vi "MATSYA GUI.vi"() -> ()   [LabVIEW 2018]
uses:
  <vilib>/picture/3D Picture Control/NI_3D Picture Control.lvlib
  179b0847-8d0b-44e4-b652-b0f693d2dd6b.vi
  a317c550-89e4-45e7-94c4-efb925d81c87.vi
  00af5911-90ac-44b2-9784-eceb848f2253.vi
  66d8c7ed-505b-4229-a511-ec78d290ed99.vi
  Host/Controls/Host Data Cluster.ctl
  Main Engine/Controls/Main Engine CPU Info.ctl
panel:
  out "AI":dbl[](array[numeric]) format="%#.6f"
  out "Data Tx/Rx 2":string
  out "output cluster":T1
  out "error out 3":errorcluster
  out "Power  Status":string
  out "USER STRING":string
  out "length":i32
  out "error in (no error) 2":errorcluster
  out "elements in queue":i32
  out "PDE_P 24 Current (A)":dbl caption="PDE_P Current (A)" format="%_3g"
  out "PDE_P 24 Voltage (V) 2":dbl caption="PDE_P Voltage (V)" format="%.1f"
  out "PDE_P 24 Voltage (V)":dbl caption="PDE_P Voltage (V)" format="%.1f"
  out "Slave":bool
  out "error out 2":errorcluster
  out "String":string
  out "Water Ingress":bool caption="AGS 1"
  out "Comm Status":bool caption="AGS 2"
  out "Temp":dbl caption="Displacement"
  out "Battery SOC":dbl caption="Displacement"
  out "CO2":dbl caption="Displacement"
  out "O2":dbl caption="Displacement"
  in  "Quit":bool caption="Power"
  in  "Mode":bool caption="Reset"
  out "Warnings/Alarms":string
  in  "Thrusters \ninterlock":bool
  out "Present Time":string caption="Present Text"
  out "Mission Start Time":string caption="Start Time Text"
  out "Dive #":dbl format="%#_2g"
  in  "Tab Control":T2(tab)
  out "Altitude":dbl(slide)=1.0 scale=0.0..90.0
  out "Depth":dbl(slide)=1.0
  out "Vertical    Speed":dbl format="%#_4g"
  out "Lateral\nSpeed":dbl format="%#.4g"
  out "Forward\nSpeed":dbl format="%#_4g"
  out "Longitude":dbl format="%#_8g"
  out "Latitude":dbl format="%#_8g"
  out "Ship\n Heading":dbl format="%#.4f"
  out "Heading":sgl
  out "Pitch":sgl
  out "Roll":sgl
  out "3D MATSYA":refnum<vi>(3d-picture)
  out "HSSS_S":T3 caption="HSSS_P" {"Oxygen_S" scale=19.0..25.0; "CO2_s" scale=0.0..5000.0; "Temp in Deg C_S" scale=0.0..100.0; "Humidity_S in %" scale=0.0..100.0; "Presssure in mbar_S" scale=800.0..1200.0}
  out "HSSS_P":T4 {"Oxygen_P" scale=19.0..25.0; "CO2_P" scale=0.0..5000.0; "Temp in Deg C_P" scale=0.0..100.0; "Humidity_P in %" scale=0.0..100.0; "Presssure in mbar_P" scale=800.0..1200.0}
  in  "HSSS_P Power":bool
  in  "Dehumidifier_S":bool
  in  "HSSS_S Power":bool
  in  "Co2 Scrubber_P":bool
  in  "Co2 Scrubber_S":bool
  in  "Dehumidifier_P":bool
  out "MBS Air Pressure 2":dbl(slide)=1.0 caption="MBS Air Pressure 1" scale=0.3..300.0
  out "Motor Water Entry":dbl
  out "HP AIR pressure 2":dbl
  out "HP AIR pressure 1":dbl
  out "HPU temp":dbl
  out "HPU Pressure":dbl
  out "MBS JB Water Entry":dbl
  in  "MBS_manual":bool
  in  "VBS SET":dbl
  in  "Trim motor enable":bool
  out "Motor temp":dbl
  out "SUB Pitch":dbl
  out "MBS Air Pressure 1":dbl(slide)=1.0 scale=0.3..300.0
  in  "VBS_Water out":bool
  in  "VBS Water In":bool
  in  "Auto Tim Enable":bool
  out "VBS Tank":dbl(slide)=1.0 scale=0.0..300.0
  in  "VBS_HPU_Enable":bool
  in  "MBS Freeboard":bool
  in  "MBS Desent":bool
  in  "Thrusters_T3":bool
  in  "T3-Signal":bool
  out "T8":T5 {"T8 Temp" format="%#.1f"; "T8 Current" format="%#_2g"; "T8 Voltage" format="%#_3g"; "T8 Speed" scale=0.0..1600.0}
  in  "T8 ctrl":dbl min=-10.0 max=10.0
  out "T6":T6 {"T6 Temp" format="%#.1f"; "T6 Current" format="%#_2g"; "T6 Voltage" format="%#_3g"; "T6 Speed" scale=0.0..1600.0}
  in  "T6 ctrl":dbl min=-10.0 max=10.0
  out "T4":T7 {"T4 Temp" format="%#.1f"; "T4 Current" format="%#_2g"; "T4 Voltage" format="%#_3g"; "T4 Speed" scale=0.0..1600.0}
  in  "T4 ctrl":dbl min=-10.0 max=10.0
  out "T2":T8 {"T2 Temp" format="%#.1f"; "T2 Current" format="%#_2g"; "T2 Voltage" format="%#_3g"; "T2 Speed" scale=0.0..1600.0}
  in  "T2 ctrl":dbl min=-10.0 max=10.0
  in  "T7 ctrl":dbl min=-10.0 max=10.0
  in  "T5 ctrl":dbl min=-10.0 max=10.0
  out "T7":T9 {"T7 Temp" format="%#.1f"; "T7 Current" format="%#_2g"; "T7 Voltage" format="%#_3g"; "T7 Speed" scale=0.0..1600.0}
  out "T5":T10 {"T5 Temp" format="%#.1f"; "T5 Current" format="%#_2g"; "T5 Voltage" format="%#_3g"; "T5 Speed" scale=0.0..1600.0}
  out "T1":T11 {"T1 Temp" format="%#.1f"; "T1 Current" format="%#_2g"; "T1 Voltage" format="%#_3g"; "T1 Speed" scale=0.0..1600.0}
  in  "T3 ctrl":dbl min=-10.0 max=10.0
  in  "T1 ctrl":dbl min=-10.0 max=10.0
  out "T3":T12 {"T3  Temp" format="%#.1f"; "T3 Current" format="%#_2g"; "T3 Voltage" format="%#_3g"; "T3 Speed" scale=0.0..1600.0}
  in  "T2Power":bool
  in  "T4Power":bool
  in  "T6Power":bool
  in  "T8Power":bool
  in  "T3Power":bool
  in  "T5Power":bool
  in  "T7Power":bool
  in  "T1Power":bool
  in  "Thrusters_T1":bool
  in  "T1-Signal":bool
  in  "Thrusters _T5":bool
  in  "T5-Signal":bool
  in  "Thrusters _T7":bool
  in  "T7-Signal":bool
  in  "Thrusters _T2":bool
  in  "T2-Signal":bool
  in  "Thrusters _T4":bool
  in  "T4-Signal":bool
  in  "Thrusters _T6":bool
  in  "T6-Signal":bool
  in  "Thrusters _T8":bool
  in  "T8-Signal":bool
  out "MB_S":T13 {"MB_S Temp (deg C)" format="%_3g"; "MB_S Power (W)" format="%_3f"; "MB_S Current (A)" format="%_3g"; "MB_S Volt (V)" scale=0.0..160.0; "MB_S SOC (%)" format="%_3g"}
  out "MB_P":T14 {"MB_P Temp (deg C)" format="%_3g"; "MB_P Power (W)" format="%_3f"; "MB_P Current (A)" format="%_3g"; "MB_P Volt (V)" scale=100.0..160.0; "MB_P SOC (%)" format="%_3g"}
  out "AUX_S":T15 {"AUX_S Temp (deg C)" format="%_3g"; "AUX_S Power (W)" format="%_3g"; "AUX_S Current (A)" format="%_3g"; "AUX_S Volt (V)" scale=0.0..60.0; "AUX_S SOC (%)" format="%_3g"}
  out "IDE_S":T16 {"IDE_S Temp (degC)" format="%_3g"; "IDE_S Current (A)" format="%_3g"; "IDE_S Voltage (V)" format="%_3g"; "IDE_S IR  (Kohm)" format="%_3f"}
  out "IDE_P":T17 {"IDE_P Temp (degC)" format="%_3g"; "IDE_P Current (A)" format="%_3g"; "IDE_P Voltage (V)" format="%_3g"; "IDE_P IR (kohm)" format="%_3f"}
  out "PDE_S":T18 {"PDE_S Current (A)" format="%_3g"; "PDE_S Temp (degC)" format="%_3g"; "PDE_S Voltage (V)" format="%.1f"; "PDE_S IR (Kohm)" format="%_3f"}
  out "PDE_P":T19 {"PDE_P Temp (degC)" format="%_3g"; "PDE_P Current (A)" format="%_3g"; "PDE_P Voltage (V)" format="%.1f"; "PDE_P IR (Kohm)" format="%_3f"}
  out "AUX_P":T20 {"AUX_P Temp (deg C)" format="%_3g"; "AUX_P Power (W)" format="%_3g"; "AUX_P Current (A)" format="%_3g"; "AUX_P Volt (V)" scale=0.0..40.0; "AUX_P SOC (%)" format="%_3g"}
  in  "HYD_OIL":bool
  in  "ALTITUDE":bool
  in  "DEPTH":bool
  in  "AB_P":bool
  in  "AB_S":bool
  in  "BATS_S":bool
  in  "TJB_S":bool
  in  "PJB_S":bool
  in  "PDE_S":bool
  in  "IDE_S":bool
  in  "PS_S":bool
  in  "MB_S":bool
  in  "PDE_148_S":bool
  in  "PDE_S":bool
  in  "IDE_S":bool
  in  "EB_S":bool
  in  "UB_S":bool
  in  "MB_P":bool
  in  "PDE_148_P":bool
  in  "PDE_P":bool
  in  "IDE_P":bool
  in  "EB_P":bool
  in  "UB_P":bool
  in  "BATS_P":bool
  in  "TJB_P":bool
  in  "PJB_P":bool
  in  "PDE_P":bool
  in  "IDE_P":bool
  in  "PS_P":bool
  out "Hyd oil":bool
  out "Depth":bool
  out "Altitude":bool
  out "PDE 148_S":bool
  out "PDE_S":bool
  out "IDE_S":bool
  out "EB_S":bool
  out "UB_S":bool
  out "AB_S":bool
  out "MB_S":bool
  out "PDE 148_P":bool
  out "PDE_P":bool
  out "IDE_P":bool
  out "EB_P":bool
  out "UB_P":bool
  out "AB_P":bool
  out "MB_P":bool
  out "TJB_S":bool
  out "PJB_S":bool
  out "PDE_S 3":bool
  out "IDE_S 3":bool
  out "PS_S":bool
  out "TJB_P":bool
  out "PJB_P":bool
  out "PDE_P 3":bool
  out "IDE_P 3":bool
  out "PS_P":bool
  out "BATS_S":bool
  out "BATS_P":bool
  in  "Dissolved O2":bool caption="LED Light S4"
  in  "Camera Controls":T21
  in  "Pan and Tilt P2":bool
  in  "148 V LED S3":bool
  in  "148 V LED S4":bool
  in  "148 V LED S1":bool
  in  "148 V LED S2":bool
  in  "LED Light S3":bool
  in  "LED Light S4":bool
  in  "HD Camera S3":bool
  in  "LED Light S2":bool
  in  "SD Camera S4":bool
  in  "HD Camera S1":bool
  in  "HD Camera S2":bool
  in  "4K camera S":bool
  in  "LED Light P3":bool
  in  "LED Light P4":bool
  in  "HD Camera P3":bool
  in  "LED Light P2":bool
  in  "SD_Camera_P4":bool
  in  "HD Camera P1":bool
  in  "HD Camera P2":bool
  in  "4K camera P":bool
  out "ROV PnT Indication":T22 {"TILT" max=120 step=2 scale=-110.0..110.0; "PAN" scale=-150.0..150.0}
  in  "PnT CTRL":T23
  in  "148 V LED P2":bool
  in  "148 V LED P1":bool
  in  "148 V LED P3":bool
  in  "148 V LED P4":bool
  in  "Pan and Tilt S":bool
  in  "Pan and Tilt P1":bool
  in  "Tab Control 2":enum32{"LED 1", "LED 2"}(tab)
  in  "led 1 Dim% (10x)":dbl(slide) caption="Dim% (10x)" min=0.0 max=5.0 step=1.0 scale=0.0..5.0
  in  "led 2 Dim% (10x)":dbl(slide) caption="Dim% (10x)" min=0.0 max=5.0 step=1.0 scale=0.0..5.0
  out "S_Depth":dbl
  out "S_Longitude":dbl
  out "S_Latitude":dbl
  out "S_Heading":dbl
  out "S_Pitch":dbl
  out "S_Roll":dbl
  in  "Dissolved Oxygen":bool
  in  "Trim System":bool
  in  "Plume Detector":bool
  out "Altitude 2":dbl format="%#_4g"
  out "Depth Sensor Sec 2":dbl format="%#_4g"
  out "Depth Sensor Pri 2":dbl format="%#_4g"
  in  "Laser Light 4":bool
  in  "Laser Light 3":bool
  in  "Laser Light 2":bool
  in  "Laser Light 1":bool
  in  "Magnetometer":bool
  in  "Heat Probe Sensor":bool
  in  "CO2 Sensor":bool
  in  "Subbottom Profiler":bool
  in  "Imaging Sonar":bool
  in  "SVP, Turbidity, pH":bool
  in  "Multibeam Sonar":bool
  out "pH":dbl format="%#_4g"
  out "Methane con":dbl format="%#_4g"
  out "Carbon Dioxide":dbl format="%#_4g"
  out "Disolved Oxygen":dbl format="%#_4g"
  in  "Altimeter":bool
  in  "Conduct & Temp":bool
  out "Turbidity":dbl format="%#_4g"
  out "Subea Temp_2":dbl format="%#_4g"
  out "Water Density":dbl format="%#_4g"
  out "Salanity":dbl format="%#_4g"
  in  "INS-DVL":bool
  in  "Depth Sensor Pri":bool
  out "Sound Velocity":dbl format="%#_4g"
  out "Conductivity":dbl format="%#_4g"
  in  "Methane_Sensor":bool
  in  "VBS":bool
  in  "MBS":bool
  out "Error Logging":string[][](table)
  in  "Data log":bool
  in  "Data Logging":dbl(slide) scale=0.0..60.0
  out "Event Logging":string[][](table)
  in  "Channel 2":u16(ring) caption="Ring"
  out "Graph 2":dbl[](graph) caption="Displacement"
  out "Graph 1":dbl[](graph) caption="Displacement"
  in  "Channel":u16(ring) caption="Ring"
  out "BAT VOL 2":dbl(slide)=1.0 scale=100.0..170.0
  out "BAT TEMP 2":dbl(slide)=1.0 scale=0.0..50.0
  out "BAT SOC 2":dbl(slide)=1.0 scale=0.0..200.0
  out "BAT CUR 2":dbl(slide)=1.0 scale=0.0..100.0
  out "BAT VOL":dbl(slide)=1.0 scale=100.0..170.0
  out "BAT TEMP":dbl(slide)=1.0 scale=0.0..50.0
  out "BAT SOC":dbl(slide)=1.0 scale=0.0..200.0
  out "BAT CUR":dbl(slide)=1.0 scale=0.0..100.0
  out "portside 50 Kwh":T24
  out "50 kwh star board":T25
  in  "read/write":bool
  in  "Enum - Menu":enum16{"Low", "Medium", "High", "Very High"}(ring)
  out "Ship Time":sgl caption="Longitude"
  out "Ship Heading":sgl caption="Longitude" format="%#_8g"
  out "Ship Latitude":sgl caption="Latitude" format="%#_9g"
  out "Ship Longitude":sgl caption="Longitude" format="%#_8g"
  in  "Read/ Write":bool
  in  "Data Sending Mode":bool
  out "Modem Ready Status":bool
  out "Data Out":string
  in  "Data Tx/Rx":string
  in  "Byte Count":u32=20
  in  "Crew Status PILOT":bool caption="PILOT"
  in  "Crew StatusCO-PILOT":bool caption="CO-PILOT"
  in  "Crew Status OBSERVER":bool caption="OBSERVER"
  out "Radio Buttons 2":enum32{"Item 0", "Item 1", "Item 2", "Item 3"}(radio)
  in  "Crew Status OBSERVER 2":bool caption="Power"
  in  "Joystick":bool
  in  "Access":bool=TRUE
  out "Quit?":bool
  out "PS_P_Comm_status":bool
  out "PS_S_Comm_Status":bool
  out "PDE_P_Comm_Status":bool
  out "PDE_S_Comm_Status":bool
  out "IDE_P_Comm_Status":bool
  out "IDE_S_Comm_Status":bool
  out "Serial":string[][](array[string])
  out "System Down?":bool
  in  "OIM RESET_S2":bool
  in  "OIM RESET _S1":bool
  in  "BATS_S":bool
  in  "OIM RESET_P2":bool
  in  "OIM RESET _P1":bool
  in  "MBS_P":bool
  in  "LED Light S1":bool
  in  "LED Light P1":bool
  out "TCP - Serial":string[][](array[string])
  in  "error In":errorcluster
  out "PS_P 2":T26
  out "IDE_P 2":T26
  out "PS_S 2":T26
  out "PDE_S 2":T26
  out "PDE_P 2":T26
  out "IDE_S 2":T26
  out "Completed Time":string caption="Elapsed Time Text"
  # "NATIONAL INSTITUTE OF OCEAN TECHNOLOGY\nManned Submersible - MATSYA 6000"
  # "Battery5\n81 Power\n82Current\n83 Pack Voltage\n84ID cell max\n85Max temperature\n86 ID Cell min\n87 Min temperature\n88 Temperature\n89 SOC\n90 SOH\n91 State Bat\n92Flags Bat\n93Fault Code\n94 Level Faults\n95Warnings"
  # "Global Data\n01 Battery Current\n02 Battery Voltage\n03 SOC\n04 SOH\n05 Mean Temperature\n06 Status Faults\n07 Status Warning\n08 Status battery\n\nSummary 10 kW modules\n09 Battery ID\n10 Max temperature\n11 Pack Max voltage\n12 battrey ID Voltgae\n13 Battery ID Min Voltage\n14 Pack Min Voltage\n15 Battery ID min\n16 ID cell Min\n17 Min Cell Voltage\n18 Battery ID Max\n19 ID cell Max\n20 Max cell voltage\n\nEach 10 kW Batteries                                                        \nBattery1\n21 Power\n22 Current\n23 Pack Voltage\n24 ID cell max\n25 Max temperature\n26 ID Cell min\n27 Min temperature\n28 Temperature\n29 SOC\n30 SOH\n31 State Bat\n32 Flags Bat\n33 Fault Code\n34 Level Faults\n35 Warnings\n\nBattery2\n36 Power\n37 Current\n38 Pack Voltage\n39 ID cell max\n40 Max temperature\n41 ID Cell min\n42 Min temperature\n43 Temperature\n44 SOC\n45 SOH\n46 State Bat\n47 Flags Bat\n48 Fault Code\n49 Level Faults\n50 Warnings\n\n\n\nBattery3\n51 Power\n52Current\n53 Pack Voltage\n54 ID cell max\n55Max temperature\n56 ID Cell min\n57 Min temperature\n58 Temperature\n59 SOC\n60 SOH\n61 State Bat\n62 Flags Bat\n63 Fault Code\n64 Level Faults\n65Warnings"
  # "Battery4\n66 Power\n67Current\n68 Pack Voltage\n69ID cell max\n70Max temperature\n71 ID Cell min\n72 Min temperature\n73 Temperature\n74 SOC\n75 SOH\n76 State Bat\n77Flags Bat\n78 Fault Code\n79 Level Faults\n80Warnings"
  # "Comm Status"
  # "N"
  # "deg"
  # "deg"
  # "E"
  # "m/s"
  # "W"
  # "m/s"
  # "m/s"
  # "S"
  # "deg"
  # "m"
  # "m"
  # "deg"
  # "MBS"
  # "VBS"
  # "TRIM"
  # "PDE_P"
  # "T_3"
  # "T_5"
  # "T_7"
  # "T_1"
  # "V"
  # "A"
  # "deg C"
  # "V"
  # "A"
  # "deg C"
  # "V"
  # "A"
  # "deg C"
  # "V"
  # "A"
  # "deg C"
  # "V"
  # "A"
  # "deg C"
  # "V"
  # "A"
  # "deg C"
  # "V"
  # "A"
  # "deg C"
  # "V"
  # "A"
  # "deg C"
  # "IDE_P"
  # "IDE_P"
  # "Insulation_S"
  # "Insulation_P"
  # "Water Ingress_S"
  # "Water Ingress_P"
  # "Underwater Imaging"
  # "deg"
  # "deg"
  # "Deg"
  # "Deg"
  # "Scientific Sensors"
  # "Sec.INS"
  # "Port side"
  # "Starboard"
  # "blow valve 1"
  # "blow valve 2"
  # "Forward"
  # "Reverse"
  # "BATTERY 50 kWh STATUS"
  # "port side"
  # "starboard side"
  # "BAT 1"
  # "BAT 4"
  # "BAT 2"
  # "BAT 3"
  # "BAT 5"
  # "CUR"
  # "VOT"
  # "ID Cell Max"
  # "Max Temp"
  # "ID Cell Min"
  # "Min Temp"
  # "Temp"
  # "SOC"
  # "SOH"
  # "BAT 6"
  # "BAT 7"
  # "BAT 8"
  # "BAT 9"
  # "BAT 10"
  # "CUR"
  # "VOT"
  # "ID Cell Max"
  # "Max Temp"
  # "ID Cell Min"
  # "Min Temp"
  # "Temp"
  # "SOC"
  # "SOH"
  # "Power Status"
  # "Crew Status"
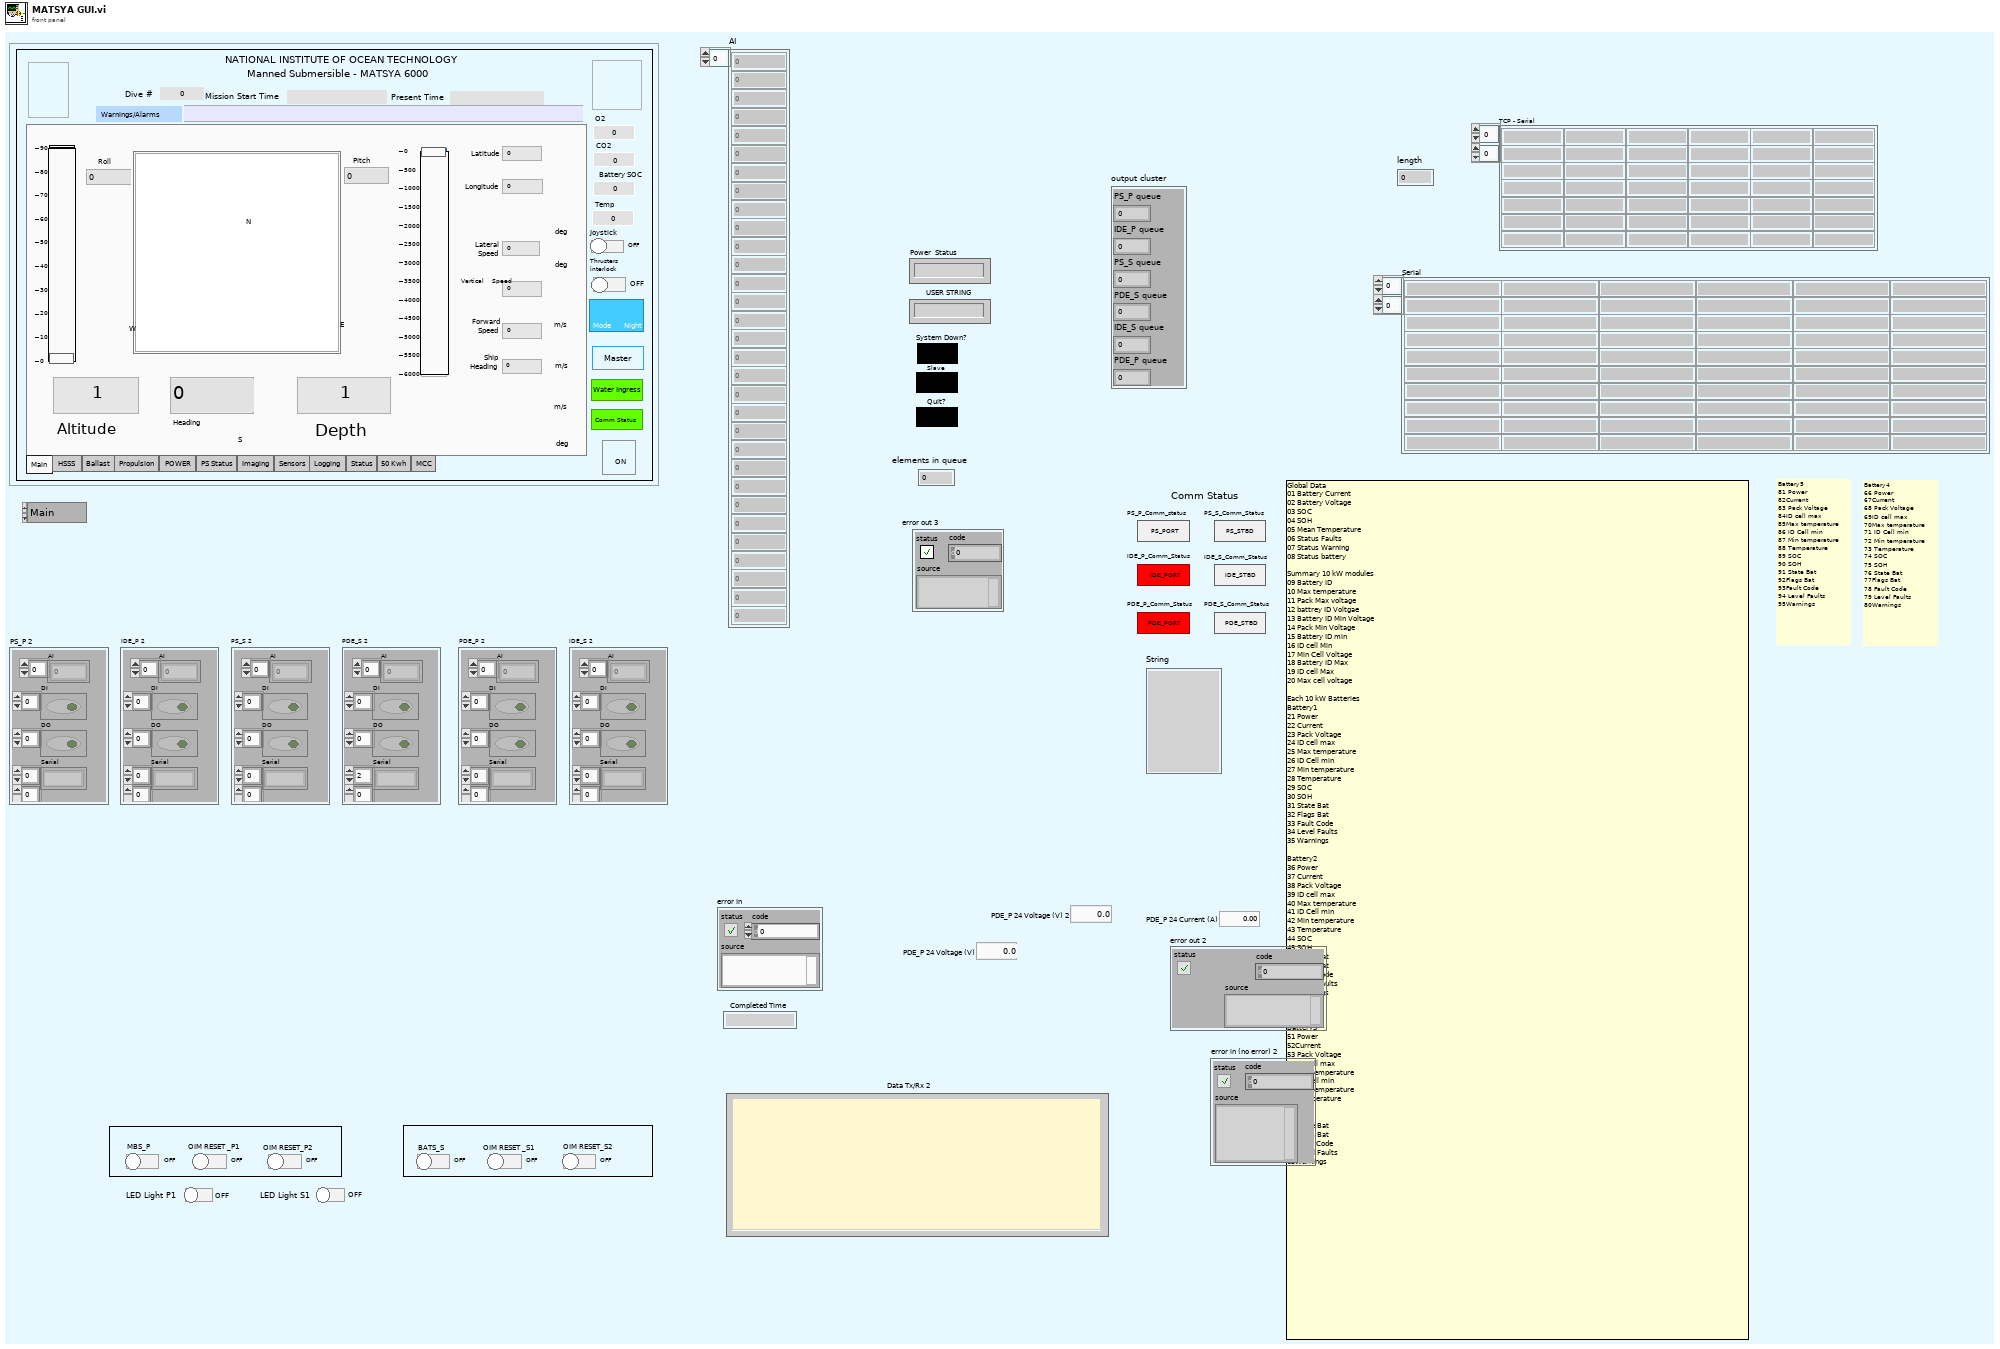
[diagram p1: front panel]
types:
  T1 = cluster{"PS_P queue":i32, "IDE_P queue":i32, "PS_S queue":i32, "PDE_S queue":i32, "IDE_S queue":i32, "PDE_P queue":i32}
  T2 = enum32{"Main", "HSSS ", "Ballast", "Propulsion", "POWER ", "PS Status", "Imaging", "Sensors", "Logging", "Status", "50 Kwh", "MCC"}
  T3 = cluster{"Presssure in mbar_S":dbl, "Humidity_S in %":dbl, "Temp in Deg C_S":dbl, "CO2_s":dbl, "Oxygen_S":dbl, "Hydrogen":dbl, "HP_B1 Pressure":dbl, "HP_B2 Pressure":dbl, "HP_B3 Pressure":dbl, "Smoke Sensor":bool, "Flame Sensor":bool, "LP_L Pressure":dbl, "Heat Sensor":bool}
  T4 = cluster{"Presssure in mbar_P":dbl, "Humidity_P in %":dbl, "Temp in Deg C_P":dbl, "CO2_P ":dbl, "Oxygen_P":dbl, "Hydrogen":dbl, "HP_B1 Pressure":dbl, "HP_B2 Pressure":dbl, "HP_B3 Pressure":dbl, "Smoke Sensor":bool, "Flame Sensor":bool, "LP_L Pressure":dbl, "Heat Sensor":bool}
  T5 = cluster{"T8 Speed":dbl, "T8 Voltage":dbl, "T8 Current":dbl, "T8 Temp":dbl}
  T6 = cluster{"T6 Speed":dbl, "T6 Voltage":dbl, "T6 Current":dbl, "T6 Temp":dbl}
  T7 = cluster{"T4 Speed":dbl, "T4 Voltage":dbl, "T4 Current":dbl, "T4 Temp":dbl}
  T8 = cluster{"T2 Speed":dbl, "T2 Voltage":dbl, "T2 Current":dbl, "T2 Temp":dbl}
  T9 = cluster{"T7 Speed":dbl, "T7 Voltage":dbl, "T7 Current":dbl, "T7 Temp":dbl}
  T10 = cluster{"T5 Speed":dbl, "T5 Voltage":dbl, "T5 Current":dbl, "T5 Temp":dbl}
  T11 = cluster{"T1 Speed":dbl, "T1 Voltage":dbl, "T1 Current":dbl, "T1 Temp":dbl}
  T12 = cluster{"T3 Speed":dbl, "T3 Voltage":dbl, "T3 Current":dbl, "T3  Temp":dbl}
  T13 = cluster{"MB_S SOC (%)":dbl, "MB_S Volt (V)":dbl, "MB_S Current (A)":dbl, "MB_S Power (W)":dbl, "MB_S Temp (deg C)":dbl}
  T14 = cluster{"MB_P SOC (%)":dbl, "MB_P Volt (V)":dbl, "MB_P Current (A)":dbl, "MB_P Power (W)":dbl, "MB_P Temp (deg C)":dbl}
  T15 = cluster{"AUX_S SOC (%)":dbl, "AUX_S Volt (V)":dbl, "AUX_S Current (A)":dbl, "AUX_S Power (W)":dbl, "AUX_S Temp (deg C)":dbl}
  T16 = cluster{"IDE_S IR  (Kohm)":dbl, "IDE_S Voltage (V)":dbl, "IDE_S Current (A)":dbl, "IDE_S Temp (degC)":dbl, "IDE_S IR Status":bool, "IDE_S Water Leak":bool}
  T17 = cluster{"IDE_P IR (kohm)":dbl, "IDE_P Voltage (V)":dbl, "IDE_P Current (A)":dbl, "IDE_P Temp (degC)":dbl, "IDE_P IR Status":bool, "IDE_P Water Leak":bool}
  T18 = cluster{"PDE_S IR (Kohm)":dbl, "PDE_S Voltage (V)":dbl, "PDE_S Temp (degC)":dbl, "PDE_S IR Status":bool, "PDE_S Water Leak":bool, "PDE_S Current (A)":dbl}
  T19 = cluster{"PDE_P IR (Kohm)":dbl, "PDE_P Voltage (V)":dbl, "PDE_P Current (A)":dbl, "PDE_P Temp (degC)":dbl, "PDE_P IR Status":bool, "PDE_P Water Leak":bool}
  T20 = cluster{"AUX_P SOC (%)":dbl, "AUX_P Volt (V)":dbl, "AUX_P Current (A)":dbl, "AUX_P Power (W)":dbl, "AUX_P Temp (deg C) ":dbl}
  T21 = cluster{"Enum - Menu":enum16{"", "Camera 2", "Camera 1"}, "ZOOM IN":bool, "ZOOM OUT":bool, "IRIS OPEN":bool, "IRIS CLOSE":bool, "ZOOM OUT 2":bool, "IRIS CLOSE 2":bool}
  T22 = cluster{"PAN":bool, "TILT":bool, "PAN":i16, "TILT":i16}
  T23 = cluster{"Pan up":bool, "manual":bool, "Tilt Right":bool, "Pan down":bool, "Tilt Left":bool, "PAN":i16, " TILT ":i16}
  T24 = cluster{"Current_1":dbl, "Current_2":dbl, "Current_3":dbl, "Current_4":dbl, "Current_5":dbl, "Voltage_1":dbl, "Voltage_2":dbl, "Voltage_3":dbl, "Voltage_4":dbl, "Voltage_5":dbl, "ID Cell Max_1":dbl, "ID Cell Max_2":dbl, "ID Cell Max_3":dbl, "ID Cell Max_4":dbl, "ID Cell Max_5":dbl, "Max Temp_1":dbl, "Max Temp_2":dbl, "Max Temp_3":dbl, "Max Temp_4":dbl, "Max Temp_5":dbl, "ID Cell Min _1":dbl, "ID Cell Min _2":dbl, "ID Cell Min _3":dbl, "ID Cell Min _4":dbl, "ID Cell Min _5":dbl, "Min Temp_1":dbl, "Min Temp_2":dbl, "Min Temp_3":dbl, "Min Temp_4":dbl, "Min Temp_5":dbl, "Temp_1":dbl, "Temp_2":dbl, "Temp_3":dbl, "Temp_4":dbl, "Temp_5":dbl, "SOC_1":dbl, "SOC_2":dbl, "SOC_3":dbl, "SOC_4":dbl, "SOC_5":dbl, "SOH_1":dbl, "SOH_2":dbl, "SOH_3":dbl, "SOH_4":dbl, "SOH_5":dbl}
  T25 = cluster{"Current_1 2":dbl, "Voltage_1 2":dbl, "ID Cell Max_1 2":dbl, "Max Temp_1 2":dbl, "ID Cell Min _1 2":dbl, "Min Temp_1 2":dbl, "Temp_1 2":dbl, "SOC_1 2":dbl, "SOH_1 2":dbl, "Current_2 2":dbl, "Voltage_2 2":dbl, "ID Cell Max_2 2":dbl, "Max Temp_2 2":dbl, "ID Cell Min _2 2":dbl, "Min Temp_2 2":dbl, "Temp_2 2":dbl, "SOC_2 2":dbl, "SOH_2 2":dbl, "Current_3 2":dbl, "Voltage_3 2":dbl, "ID Cell Max_3 2":dbl, "Max Temp_3 2":dbl, "ID Cell Min _3 2":dbl, "Min Temp_3 2":dbl, "Temp_3 2":dbl, "SOC_3 2":dbl, "SOH_3 2":dbl, "Current_4 2":dbl, "Voltage_4 2":dbl, "ID Cell Max_4 2":dbl, "Max Temp_4 2":dbl, "ID Cell Min _4 2":dbl, "Min Temp_4 2":dbl, "Temp_4 2":dbl, "SOC_4 2":dbl, "SOH_4 2":dbl, "Current_5 2":dbl, "Voltage_5 2":dbl, "ID Cell Max_5 2":dbl, "Max Temp_5 2":dbl, "ID Cell Min _5 2":dbl, "Min Temp_5 2":dbl, "Temp_5 2":dbl, "SOC_5 2":dbl, "SOH_5 2":dbl}
  T26 = typedef "Host Data Cluster.ctl" = cluster{"AI":dbl[], "DI":bool[], "DO":bool[], "Serial":string[][], "CPU":T27, "Stop":bool, "DO Channel":string[]}
  T27 = typedef "Main Engine CPU Info.ctl" = cluster{"Total Load":u32[], "Interrupt Load":u32[], "Total Physical":dbl, "Free Physical":dbl, "Primary Disk Capacity":dbl, "Primary Disk Free":dbl}
  T28 = cluster{"Presssure in mbar":dbl, "Humidity_P in %":dbl, "Temp in Deg C":dbl, "CO2 ":dbl, "Oxygen_P":dbl, "Hydrogen":dbl, "HP_B1 Pressure":dbl, "HP_B2 Pressure":dbl, "HP_B3 Pressure":dbl, "Smoke Sensor":bool, "Flame Sensor":bool, "LP_L Pressure":dbl, "Heat Sensor":bool}
  T29 = enum16{"TCPIP acoustic stop", "read write state", "command mode", "Disable Extended Notification", "bitrate", "initialization", "Int Power Status"}
  T30 = typedef "Host - GUI Data Cluster.ctl" = cluster{"VI References":refnum<vi>[], "Addresses":string[], "Pilot":bool, "DO Data":cluster{"Names":string[], "Data":bool[]}[], "Access Restricted?":bool, "Pilot Control References":refnum<vi>[], "CoPilot Control References":refnum<vi>[], "cRIO Config":cluster{"AI":T31, "DI":T35, "DO":T35, "Async":T38}[], "datalog Q":refnum<queue>, "PS_P":T26, "PS_S":T26, "IDE_P":T26, "IDE_S":T26, "PDE_P":T26, "PDE_S":T26, "GUI References":cluster{"Control Names":string[], "Control References":refnum<vi>[]}, "GUI Data":string[][], "TCP - Serial":string[][], "TCP-Serial Q":refnum<queue>, "TCP Serial Ref":refnum<vi>[], "Data Sets":dbl[][], "Last Data":dbl[], "Alarm Data":cluster{"Alarm Value":dbl, "Data Index":i32, "DO target Index":i32, "DO Index":i32, "DI target Index":i32, "DI Index":i32}[], "DI Data":cluster{bool[]}[], "Ack Data":cluster{"Alarm Value":dbl, "Data Index":i32, "DO target Index":i32, "DO Index":i32, "DI target Index":i32, "DI Index":i32}[], "Buzzer Data":cluster{"Alarm Value":dbl, "Data Index":i32, "DO target Index":i32, "DO Index":i32, "DI target Index":i32, "DI Index":i32}[], "Pilot DO":cluster{"Data":i32[]}[], "Co-Pilot DO":cluster{"Data":i32[]}[], "System Down?":bool, "Log Data":dbl[], "Update Array":i32[][], "MCC Data Log":dbl[], "MCC Data Not":refnum<notifier>, "Thruster control":refnum<vi>[], "waga notifier out":refnum<notifier>, "Wago  log":sgl[], "Thruster Cont":dbl[], "Cam Cont":bool[], "PDE_P TH Cont":cluster{"COM 10":dbl, "COM 11":dbl, "COM 12":dbl, "COM 13":dbl}, "PDE_S TH Cont":cluster{"COM 10":dbl, "COM 11":dbl, "COM 12":dbl, "COM 13":dbl}}
  T31 = typedef "AO JSON Data Cluster.ctl" = cluster{"Interface":string, "Interface Data":T32}
  T32 = typedef "AO Interface Data Cluster.ctl" = cluster{"Command":string, "SubCmd":string, "Data":T33[], "Timing":T34}
  T33 = typedef "AO Channel Configuration Cluster.ctl" = cluster{"Channel":string, "Min Value":dbl, "Max Value":dbl, "Type":string, "Terminal Configure":u16, "Dynamic":u8, "Dyn Type":string, "Data":dbl[], "File Name":string, "Column":i32, "Frequency":dbl}
  T34 = typedef "AO Timing Cluster.ctl" = cluster{"samples per channel":i32, "sample mode":i32, "rate":dbl}
  T35 = typedef "DIO Configuration cluster.ctl" = cluster{"Interface":string, "Interface Data":T36}
  T36 = typedef "DIO Interface Data.ctl" = cluster{"Command":string, "SubCmd":string, "Frequency":u16, "Data":T37[]}
  T37 = typedef "Digital Dynamic Cluster.ctl" = cluster{"Channel":string, "Data":u8[]}
  T38 = typedef "Async JSON Cluster.ctl" = cluster{"Interface":string, "Interface Data":T39}
  T39 = typedef "Async Interface Data Cluster.ctl" = cluster{"Command":string, "SubCmd":string, "Data":T40[]}
  T40 = typedef "Async Serial Configuration Cluster.ctl" = cluster{"Port":string, "Minor Frame Freq":u16, "Minor Frame Count":u16, "Frame Info":T41[], "Sensor Type":u16, "OIM Address":u16}
  T41 = typedef "Async Frame Info Cluster.ctl" = cluster{"Frame ID":u16, "Message Info":T42[]}
  T42 = typedef "Async Message Info Cluster.ctl" = cluster{"Message":u8[], "Message Name":string}
  T43 = enum8{"Enabled", "Disabled", "Disabled and Grayed Out"}
  T44 = cluster{"TIME":sgl, "LATITUDE":sgl, "LONGITUDE":sgl, "HEADING":sgl, "Acoustic data":i32}
  T45 = cluster{"Thrusters_T1":bool, "Thrusters _T2":bool, "Thrusters_T3":bool, "Thrusters _T4":bool, "Thrusters _T5":bool, "Thrusters _T6":bool, "Thrusters _T7":bool, "Thrusters _T8":bool}
  T46 = cluster{"T1 - Signal":bool, "T2 - Signal":bool, "T3 - Signal":bool, "T4 - Signal":bool, "T5 - Signal":bool, "T6 - Signal":bool, "T7 - Signal":bool, "T8 - Signal":bool}
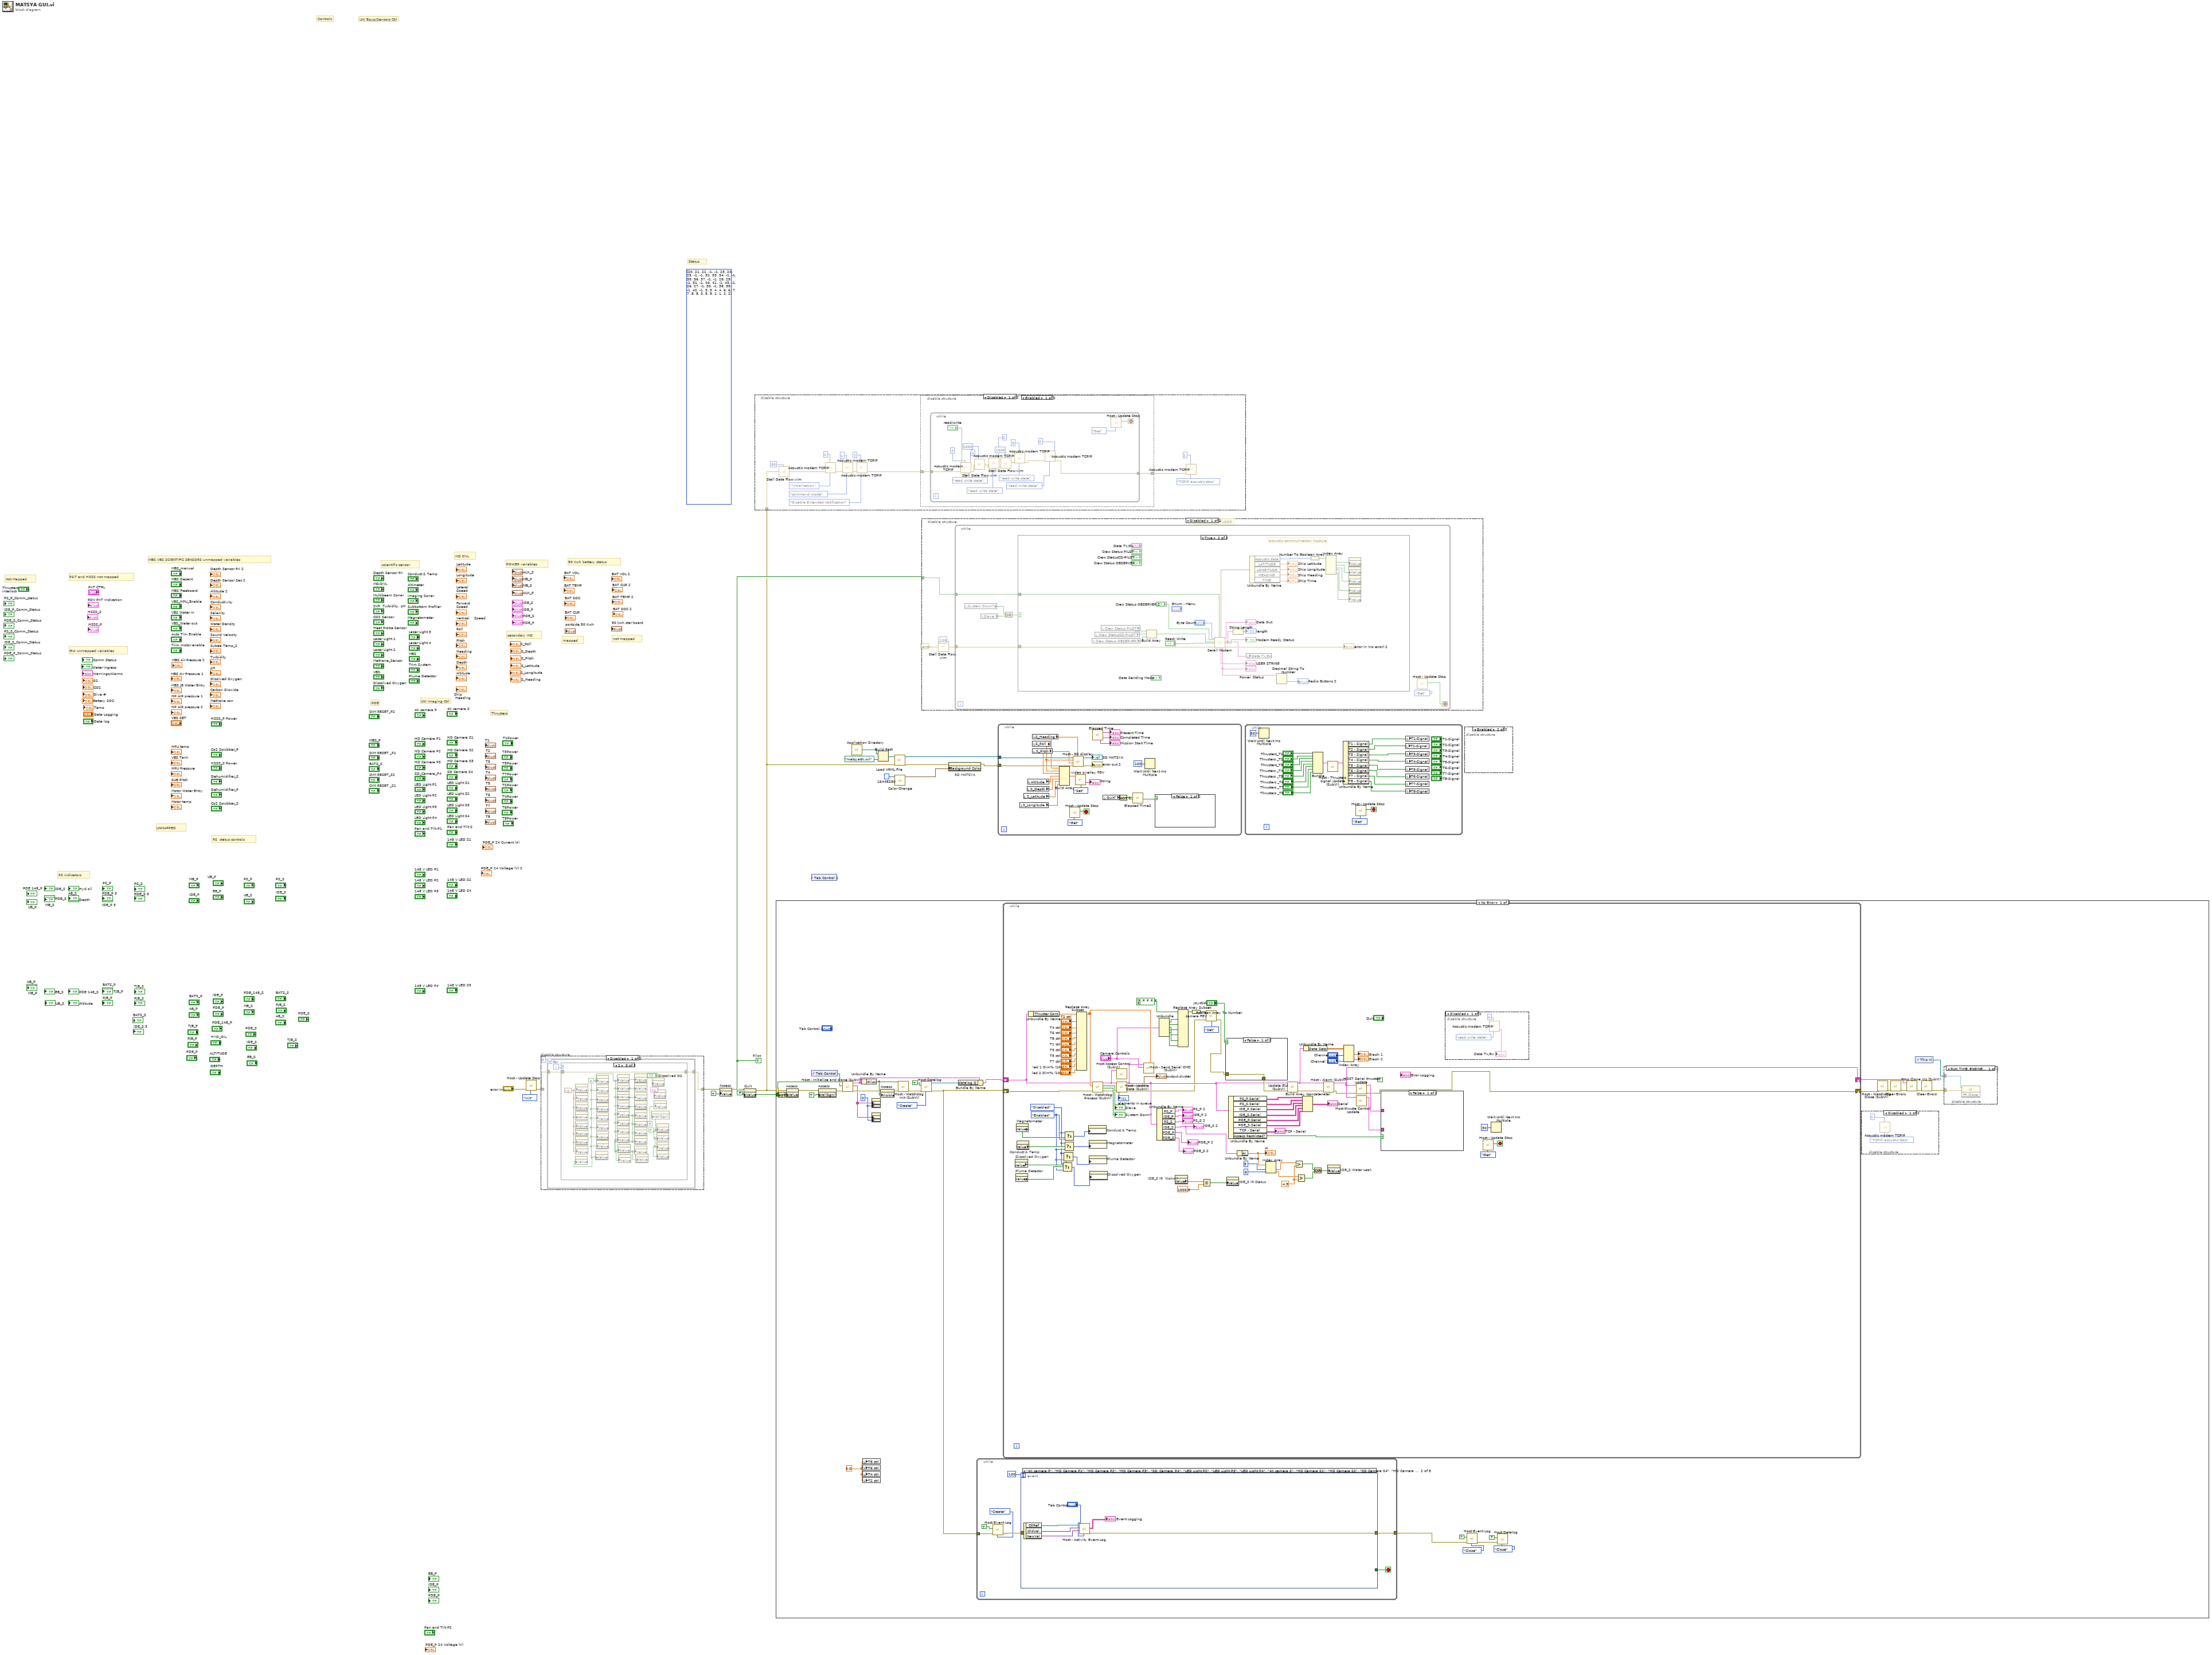
[diagram p0: block diagram]
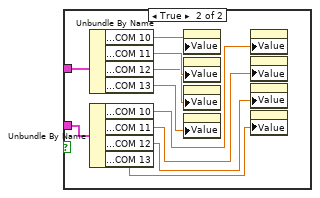
[diagram p8: hidden frame]
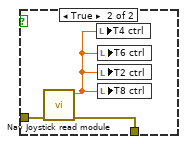
[diagram p9: hidden frame]
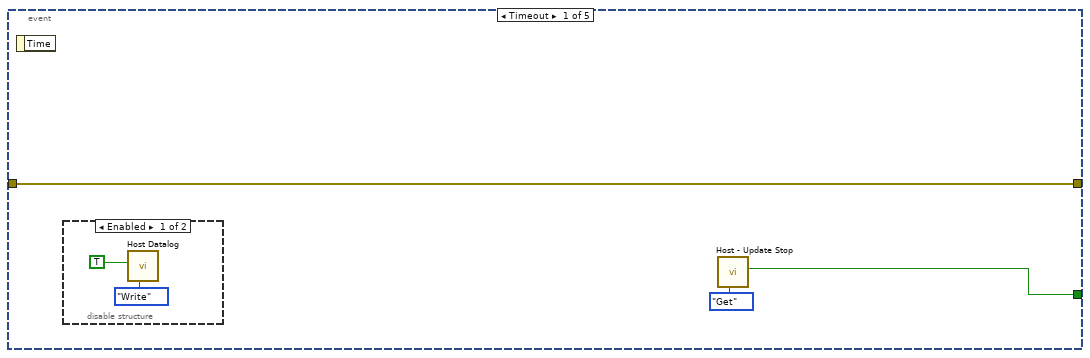
[diagram p10: hidden frame]
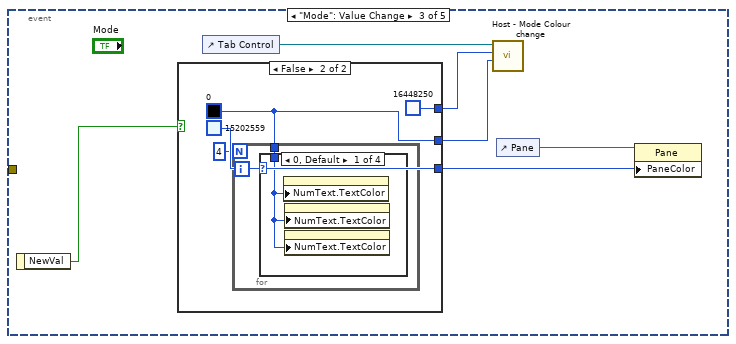
[diagram p12: hidden frame]
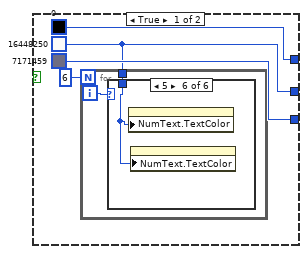
[diagram p13: hidden frame]
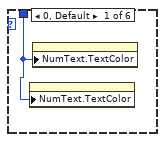
[diagram p14: hidden frame]
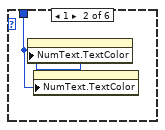
[diagram p15: hidden frame]
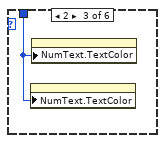
[diagram p16: hidden frame]
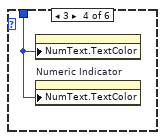
[diagram p17: hidden frame]
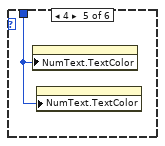
[diagram p18: hidden frame]
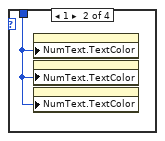
[diagram p19: hidden frame]
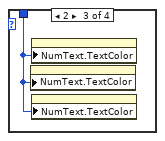
[diagram p20: hidden frame]
diagram:
  (unwired) i32[] [20, 21, 22, -1, -1, 23, 24, 25, -1, -1, 32, 33, 34, -1, -1, 35, 36, 37, -1, -1, 28, 29, -1, 31, -1, 40, 41, -1, 43, -1, 26, 27, -1, 30, -1, 38, 39, -1, 42, -1, 3, 3, 4, 4, 6, 6, 7, 7, 8, 8, 0, 5, 9, 1, 1, 2, 2]
  w5 = TRUE  # Pilot
  # "UNMAPPED"
  # "PS Indicators"
  # "Not Mapped"
  # "not mapped"
  # "mapped"
  # "P&T and HSSS not mapped"
  # "50 Kwh battery status"
  # "POWER variables"
  # "secondary INS"
  # "MBS VBS SCIENTIFIC SENSORS unmapped variables"
  # "PS  status controls"
  # "GUI unmapped variables"
  # "INS DVL"
  # "scientific sensor"
  # "PDE"
  # "Thrusters"
  # "Status"
  # "UW Imaging Ctrl"
  # "UW Equp/Sensors Ctrl"
  # "Controls"
  n1 = call "Host - Update Stop.vi"("Operation"=enum16{"Init", "Get", "Set"}."Init", "error in"="error In") -> ("error out"=w8:errorcluster)  [unwired: 8 in, 1 out]
  n2 = disable-structure shown="Disabled" {
    disable-tunnel: w8 -> [w19 w38]
    disable-tunnel: [w18 w39] -> w7
    frame Disabled {
      n3 = for {
        N: 3 -> [_]
        tunnel: w19 -> [w22]
        tunnel: [w21] -> w18
        i -> [w23]
        n4 = case shown="2" w23 {
          tunnel: w22 -> [w27 w31 w35]
          tunnel: [w27 w31 w35] -> w21
          frame 0, Default {
            w26 = string[][] [] ("Event Logging")
            w25 = 0.0 ("HPU temp")
            n5 = property on="MBS Air Pressure 1" class="Slide (strict)"(error in=w27, "Value"=w25) -> (error out=w28:errorcluster)  [unwired: 1 in, 1 out]
            n6 = property on="SUB Pitch" class="DigNum (strict)"(error in=w27, "Value"=w25) -> ()  [unwired: 1 in, 2 out]
            n7 = property on="MBS JB Water Entry" class="DigNum (strict)"(error in=w27, "Value"=w25) -> ()  [unwired: 1 in, 2 out]
            n8 = property on="HP AIR pressure 1" class="DigNum (strict)"(error in=w27, "Value"=w25) -> ()  [unwired: 1 in, 2 out]
            n9 = property on="VBS SET" class="DigNum (strict)"(error in=w27, "Value"=w25) -> ()  [unwired: 1 in, 2 out]
            n10 = local write "Event Logging"(w26) -> ()
            n11 = property on="HPU temp" class="DigNum (strict)"(error in=w28, "Value"=w25) -> ()  [unwired: 1 in, 2 out]
            n12 = property on="Motor temp" class="DigNum (strict)"(error in=w28, "Value"=w25) -> ()  [unwired: 1 in, 2 out]
            n13 = property on="HP AIR pressure 2" class="DigNum (strict)"("Value"=w25) -> ()  [unwired: 2 in, 2 out]
            n14 = property on="Motor Water Entry" class="DigNum (strict)"("Value"=w25) -> ()  [unwired: 2 in, 2 out]
            n15 = property on="VBS Tank" class="Slide (strict)"("Value"=w25) -> ()  [unwired: 2 in, 2 out]
            n16 = property on="HPU Pressure" class="DigNum (strict)"("Value"=w25) -> ()  [unwired: 2 in, 2 out]
            n17 = property on="MBS Air Pressure 2" class="Slide (strict)"("Value"=w25) -> ()  [unwired: 2 in, 2 out]
            n18 = property on="Water Density" class="DigNum (strict)"("Value"=w25) -> ()  [unwired: 2 in, 2 out]
            n19 = property on="Sound Velocity" class="DigNum (strict)"("Value"=w25) -> ()  [unwired: 2 in, 2 out]
            n20 = property on="Sound Velocity" class="DigNum (strict)"("Value"=w25) -> ()  [unwired: 2 in, 2 out]
            n21 = property on="pH" class="DigNum (strict)"("Value"=w25) -> ()  [unwired: 2 in, 2 out]
            n22 = property on="Disolved Oxygen" class="DigNum (strict)"("Value"=w25) -> ()  [unwired: 2 in, 2 out]
            n23 = property on="Carbon Dioxide" class="DigNum (strict)"("Value"=w25) -> ()  [unwired: 2 in, 2 out]
            n24 = property on="Event Logging" class="Tbl (strict)"("Value"=w26) -> ()  [unwired: 2 in, 2 out]
            n25 = property on="Methane con" class="DigNum (strict)"("Value"=w25) -> ()  [unwired: 2 in, 2 out]
            n26 = property on="Depth Sensor Pri 2" class="DigNum (strict)"("Value"=w25) -> ()  [unwired: 2 in, 2 out]
            n27 = property on="Depth Sensor Sec 2" class="DigNum (strict)"("Value"=w25) -> ()  [unwired: 2 in, 2 out]
            n28 = property on="Altitude 2" class="DigNum (strict)"("Value"=w25) -> ()  [unwired: 2 in, 2 out]
            n29 = property on="Conductivity" class="DigNum (strict)"("Value"=w25) -> ()  [unwired: 2 in, 2 out]
            n30 = property on="Salanity" class="DigNum (strict)"("Value"=w25) -> ()  [unwired: 2 in, 2 out]
            n31 = property on="Turbidity" class="DigNum (strict)"("Value"=w25) -> ()  [unwired: 2 in, 2 out]
            n32 = property on="Error Logging" class="Tbl (strict)"("Value"=w26) -> ()  [unwired: 2 in, 2 out]
            n33 = property on="S_Depth" class="DigNum (strict)"("Value"=w25) -> ()  [unwired: 2 in, 2 out]
            n34 = property on="Tab Control" class="TabCtl (strict)"("Value"=T2."Main" ("Tab Control")) -> ()  [unwired: 2 in, 2 out]
          }
          frame 1 {
            w29 = FALSE ("Dehumidifier_S")
            n35 = property on="Dehumidifier_S" class="Bool (strict)"("Value"=w29) -> ()  [unwired: 2 in, 2 out]
            n36 = property on="Co2 Scrubber_S" class="Bool (strict)"("Value"=w29) -> ()  [unwired: 2 in, 2 out]
            n37 = property on="HSSS_P Power" class="Bool (strict)"("Value"=w29) -> ()  [unwired: 2 in, 2 out]
            n38 = property on="Co2 Scrubber_P" class="Bool (strict)"("Value"=w29) -> ()  [unwired: 2 in, 2 out]
            n39 = property on="Dehumidifier_P" class="Bool (strict)"("Value"=w29) -> ()  [unwired: 2 in, 2 out]
            n40 = property on="HSSS_S Power" class="Bool (strict)"("Value"=w29) -> ()  [unwired: 2 in, 2 out]
            n41 = local write "Warnings/Alarms"("" ("Warnings/Alarms")) -> ()
            n42 = local write "T2-Signal"(w29) -> ()
            n43 = local write "T1-Signal"(w29) -> ()
            n44 = local write "T3-Signal"(w29) -> ()
            n45 = local write "T4-Signal"(w29) -> ()
            n46 = local write "T5-Signal"(w29) -> ()
            n47 = local write "T6-Signal"(w29) -> ()
            n48 = local write "T7-Signal"(w29) -> ()
            n49 = local write "T8-Signal"(w29) -> ()
            n50 = property on="HD Camera S3" class="Bool (strict)"("Value"=w29) -> ()  [unwired: 2 in, 2 out]
            n51 = property on="SD Camera S4" class="Bool (strict)"("Value"=w29) -> ()  [unwired: 2 in, 2 out]
            n52 = property on="LED Light S1" class="Bool (strict)"("Value"=w29) -> ()  [unwired: 2 in, 2 out]
            n53 = property on="HD Camera S2" class="Bool (strict)"("Value"=w29) -> ()  [unwired: 2 in, 2 out]
            n54 = property on="148 V LED S3" class="Bool (strict)"("Value"=w29) -> ()  [unwired: 2 in, 2 out]
            n55 = property on="148 V LED P4" class="Bool (strict)"("Value"=w29) -> ()  [unwired: 2 in, 2 out]
            n56 = property on="148 V LED S2" class="Bool (strict)"("Value"=w29) -> ()  [unwired: 2 in, 2 out]
            n57 = property on="148 V LED S1" class="Bool (strict)"("Value"=w29) -> ()  [unwired: 2 in, 2 out]
            n58 = property on="Magnetometer" class="Bool (strict)"("Value"=w29) -> ()  [unwired: 2 in, 2 out]
            n59 = property on="Laser Light 3" class="Bool (strict)"("Value"=w29) -> ()  [unwired: 2 in, 2 out]
            n60 = property on="Laser Light 4" class="Bool (strict)"("Value"=w29) -> ()  [unwired: 2 in, 2 out]
            n61 = property on="MBS" class="Bool (strict)"("Value"=w29) -> ()  [unwired: 2 in, 2 out]
            n62 = property on="Trim System" class="Bool (strict)"("Value"=w29) -> ()  [unwired: 2 in, 2 out]
            n63 = property on="Plume Detector" class="Bool (strict)"("Value"=w29) -> ()  [unwired: 2 in, 2 out]
            n64 = property on="Laser Light 2" class="Bool (strict)"("Value"=w29) -> ()  [unwired: 2 in, 2 out]
            n65 = property on="Subbottom Profiler" class="Bool (strict)"("Value"=w29) -> ()  [unwired: 2 in, 2 out]
            n66 = property on="Conduct & Temp" class="Bool (strict)"("Value"=w29) -> ()  [unwired: 2 in, 2 out]
            n67 = property on="Altimeter" class="Bool (strict)"("Value"=w29) -> ()  [unwired: 2 in, 2 out]
            n68 = property on="Imaging Sonar" class="Bool (strict)"("Value"=w29) -> ()  [unwired: 2 in, 2 out]
            n69 = property on="LED Light P2" class="Bool (strict)"("Value"=w29) -> ()  [unwired: 2 in, 2 out]
            n70 = property on="Methane_Sensor" class="Bool (strict)"("Value"=w29) -> ()  [unwired: 2 in, 2 out]
            n71 = property on="VBS" class="Bool (strict)"("Value"=w29) -> ()  [unwired: 2 in, 2 out]
            n72 = property on="Dissolved Oxygen" class="Bool (strict)"("Value"=w29) -> ()  [unwired: 2 in, 2 out]
          }
          frame 2 {
            w33 = FALSE ("Value (Signaling)")
            w36 = T28 {"Presssure in mbar"=0.0, "Humidity_P in %"=0.0, "Temp in Deg C"=0.0, "CO2 "=0.0, "Oxygen_P"=0.0, "Hydrogen"=0.0, "HP_B1 Pressure"=0.0, "HP_B2 Pressure"=0.0, "HP_B3 Pressure"=0.0, "Smoke Sensor"=FALSE, "Flame Sensor"=FALSE, "LP_L Pressure"=0.0, "Heat Sensor"=FALSE} ("HSSS_P")
            w32 = FALSE ("148 V LED P1")
            w37 = T11 {"T1 Speed"=0.0, "T1 Voltage"=0.0, "T1 Current"=0.0, "T1 Temp"=0.0} ("T1")
            n73 = property on="T7Power" class="Bool (strict)"("Value"=w32) -> ()  [unwired: 2 in, 2 out]
            n74 = property on="T1" class="Clust (strict)"("Value"=w37) -> ()  [unwired: 2 in, 2 out]
            n75 = property on="T2" class="Clust (strict)"("Value"=w37) -> ()  [unwired: 2 in, 2 out]
            n76 = property on="T3" class="Clust (strict)"("Value"=w37) -> ()  [unwired: 2 in, 2 out]
            n77 = property on="T4" class="Clust (strict)"("Value"=w37) -> ()  [unwired: 2 in, 2 out]
            n78 = property on="T5" class="Clust (strict)"("Value"=w37) -> ()  [unwired: 2 in, 2 out]
            n79 = property on="T6" class="Clust (strict)"("Value"=w37) -> ()  [unwired: 2 in, 2 out]
            n80 = property on="T7" class="Clust (strict)"("Value"=w37) -> ()  [unwired: 2 in, 2 out]
            n81 = property on="T8" class="Clust (strict)"("Value"=w37) -> ()  [unwired: 2 in, 2 out]
            n82 = property on="T1Power" class="Bool (strict)"("Value"=w32) -> ()  [unwired: 2 in, 2 out]
            n83 = property on="148 V LED P1" class="Bool (strict)"("Value"=w32) -> ()  [unwired: 2 in, 2 out]
            n84 = property on="LED Light S2" class="Bool (strict)"("Value"=w32) -> ()  [unwired: 2 in, 2 out]
            n85 = property on="HD Camera S1" class="Bool (strict)"("Value"=w32) -> ()  [unwired: 2 in, 2 out]
            n86 = property on="LED Light S3" class="Bool (strict)"("Value"=w32) -> ()  [unwired: 2 in, 2 out]
            n87 = property on="LED Light S4" class="Bool (strict)"("Value"=w32) -> ()  [unwired: 2 in, 2 out]
            n88 = property on="Pan and Tilt S" class="Bool (strict)"("Value"=w32) -> ()  [unwired: 2 in, 2 out]
            n89 = property on="148 V LED P2" class="Bool (strict)"("Value"=w32) -> ()  [unwired: 2 in, 2 out]
            n90 = property on="148 V LED P3" class="Bool (strict)"("Value"=w32) -> ()  [unwired: 2 in, 2 out]
            n91 = property on="4K camera P" class="Bool (strict)"("Value"=w32) -> ()  [unwired: 2 in, 2 out]
            n92 = property on="HD Camera P1" class="Bool (strict)"("Value"=w32) -> ()  [unwired: 2 in, 2 out]
            n93 = property on="HD Camera P2" class="Bool (strict)"("Value"=w32) -> ()  [unwired: 2 in, 2 out]
            n94 = property on="HD Camera P3" class="Bool (strict)"("Value"=w32) -> ()  [unwired: 2 in, 2 out]
            n95 = property on="SD_Camera_P4" class="Bool (strict)"("Value"=w32) -> ()  [unwired: 2 in, 2 out]
            n96 = property on="4K camera S" class="Bool (strict)"("Value"=w32) -> ()  [unwired: 2 in, 2 out]
            n97 = property on="LED Light P1" class="Bool (strict)"("Value"=w32) -> ()  [unwired: 2 in, 2 out]
            n98 = property on="148 V LED S4" class="Bool (strict)"("Value"=w32) -> ()  [unwired: 2 in, 2 out]
            n99 = property on="INS-DVL" class="Bool (strict)"("Value"=w32) -> ()  [unwired: 2 in, 2 out]
            n100 = property on="T3Power" class="Bool (strict)"("Value"=w32) -> ()  [unwired: 2 in, 2 out]
            n101 = property on="Multibeam Sonar" class="Bool (strict)"("Value"=w32) -> ()  [unwired: 2 in, 2 out]
            n102 = property on="SVP, Turbidity, pH" class="Bool (strict)"("Value"=w32) -> ()  [unwired: 2 in, 2 out]
            n103 = property on="CO2 Sensor" class="Bool (strict)"("Value"=w32) -> ()  [unwired: 2 in, 2 out]
            n104 = property on="Heat Probe Sensor" class="Bool (strict)"("Value"=w32) -> ()  [unwired: 2 in, 2 out]
            n105 = property on="Laser Light 1" class="Bool (strict)"("Value"=w32) -> ()  [unwired: 2 in, 2 out]
            n106 = property on="LED Light P3" class="Bool (strict)"("Value"=w32) -> ()  [unwired: 2 in, 2 out]
            n107 = property on="LED Light P4" class="Bool (strict)"("Value"=w32) -> ()  [unwired: 2 in, 2 out]
            n108 = property on="Pan and Tilt P1" class="Bool (strict)"("Value"=w32) -> ()  [unwired: 2 in, 2 out]
            n109 = property on="Depth Sensor Pri" class="Bool (strict)"("Value"=w32) -> ()  [unwired: 2 in, 2 out]
            n110 = property on="T5Power" class="Bool (strict)"("Value"=w32) -> ()  [unwired: 2 in, 2 out]
            n111 = property on="Mode" class="Bool (strict)"("Val(Sgnl)"=w33) -> ()  [unwired: 2 in, 2 out]
            n112 = property on="HSSS_S" class="Clust (strict)"("Value"=w36) -> ()  [unwired: 2 in, 2 out]
            n113 = property on="HSSS_P" class="Clust (strict)"("Value"=w36) -> ()  [unwired: 2 in, 2 out]
            n114 = property on="Quit?" class="Bool (strict)"("Value"=FALSE ("Quit?")) -> ()  [unwired: 2 in, 2 out]
            n115 = property on="T2Power" class="Bool (strict)"("Value"=w33) -> ()  [unwired: 2 in, 2 out]
            n116 = property on="T4Power" class="Bool (strict)"("Value"=w33) -> ()  [unwired: 2 in, 2 out]
            n117 = property on="T6Power" class="Bool (strict)"("Value"=w33) -> ()  [unwired: 2 in, 2 out]
            n118 = property on="T8Power" class="Bool (strict)"("Value"=w33) -> ()  [unwired: 2 in, 2 out]
          }
        }
      }
    }
    frame Enabled {
      n119 = control-ref of="This VI"() -> (w40:refnum<vi>)
      n120 = invoke class="VI" method="Default Vals.Reinit All"(reference=w40, error in=w38) -> (error out=w39:errorcluster)  [unwired: 1 in, 2 out]
    }
  }
  n121 = property on="Access" class="Bool (strict)"(error in=w7, "Value"=TRUE ("Access")) -> (error out=w2:errorcluster)  [unwired: 1 in, 1 out]
  n122 = property on="Quit" class="Bool (strict)"(error in=w2, "Value"=FALSE ("Quit")) -> (error out=w1:errorcluster)  [unwired: 1 in, 1 out]
  n123 = disable-structure shown="Disabled" {
    disable-tunnel: w1 -> [w42 _]
    frame Disabled {
      n124 = call "Stall Data Flow.vim"("value in"=w42, "milliseconds to wait"=u32 50) -> ("value out"=w41:errorcluster)  [unwired: 1 out]
      n125 = call "Acoustic modem TCPIP.vi"("Enum"=T29."initialization", "lOPP COUNT"=1, "error in (no error)"=w41) -> ("error out"=w49:errorcluster)  [unwired: 6 in, 2 out]
      n126 = call "Acoustic modem TCPIP.vi"("Enum"=T29."command mode", "lOPP COUNT"=1, "error in (no error)"=w49) -> ("error out"=w48:errorcluster)  [unwired: 6 in, 2 out]
      n127 = call "Acoustic modem TCPIP.vi"("Enum"=T29."Disable Extended Notification", "lOPP COUNT"=1, "error in (no error)"=w48) -> ("error out"=w47:errorcluster)  [unwired: 6 in, 2 out]
      n128 = disable-structure shown="Enabled" {
        disable-tunnel: w47 -> [w57 _]
        disable-tunnel: [w56 _] -> w44
        frame Enabled {
          n129 = while {
            tunnel: w57 -> [w77]
            tunnel: [w72] -> w56
            stop <- w75 stop-if-true
            n130 = call "Acoustic modem TCPIP.vi"("strings num"=1, "Enum"=T29."read write state", "lOPP COUNT"=4, "error in (no error)"=w77, "Read/Write"="read/write") -> ("error out"=w63:errorcluster)  [unwired: 4 in, 2 out]
            n131 = call "Stall Data Flow.vim"("value in"=w63, "milliseconds to wait"=u32 1000) -> ("value out"=w64:errorcluster)  [unwired: 1 out]
            n132 = call "Acoustic modem TCPIP.vi"("strings num"=2, "Enum"=T29."read write state", "error in (no error)"=w64) -> ("error out"=w61:errorcluster)  [unwired: 6 in, 2 out]
            n133 = call "Stall Data Flow.vim"("value in"=w61, "milliseconds to wait"=u32 1000) -> ("value out"=w60:errorcluster)  [unwired: 1 out]
            n134 = call "Acoustic modem TCPIP.vi"("Enum"=T29."read write state", "lOPP COUNT"=3, "error in (no error)"=w60) -> ("error out"=w58:errorcluster)  [unwired: 6 in, 2 out]
            n135 = call "Acoustic modem TCPIP.vi"("strings num"=4, "Enum"=T29."read write state", "error in (no error)"=w58) -> ("error out"=w72:errorcluster)  [unwired: 6 in, 2 out]
            n136 = call "Host - Update Stop.vi"("Operation"=enum16{"Init", "Get", "Set"}."Get") -> ("Stop?"=w75:bool)  [unwired: 9 in, 1 out]
          }
        }
        frame Disabled {
        }
      }
      n137 = call "Acoustic modem TCPIP.vi"("Enum"=T29."TCPIP acoustic stop", "lOPP COUNT"=1, "error in (no error)"=w44) -> ()  [unwired: 6 in, 3 out]
    }
    frame Enabled {
    }
  }
  n138 = case shown="No Error" w1 {
    selector: w1 -> [w83 _]
    tunnel: w5 -> [w85 _]
    frame No Error {
      w98 = 0.0 ("T8 ctrl")
      w99 = 0
      n139 = Not(x=w85) -> (.not. x?=w91:bool)
      n140 = property on="Access" class="Bool (strict)"(error in=w83, "Value"=w91) -> (error out=w93:errorcluster)  [unwired: 1 in, 1 out]
      n141 = control-ref of="Tab Control"() -> (w84:refnum<vi>)
      n142 = property on="Access" class="Bool (strict)"(error in=w93, "Val(Sgnl)"=TRUE ("Value (Signaling)")) -> (error out=w82:errorcluster)  [unwired: 1 in, 1 out]
      n143 = call "Host - Initialise and clone (SubVI).vi"("Pilot"=w85, "error in"=w82, "Tab Reference"=w84) -> ("error out"=w106:errorcluster, "Control names"=w100:string[], "Data Cluster"=w107:T30)  [unwired: 6 in]
      n144 = Unbundle By Name(w107) -> ("Pilot"=w104:bool)
      n145 = local write "T8 ctrl"(w98) -> ()
      n146 = local write "T6 ctrl"(w98) -> ()
      n147 = local write "T4 ctrl"(w98) -> ()
      n148 = local write "T2 ctrl"(w98) -> ()
      n149 = property on="Channel" class="Ring (strict)"("Strings []"=w100, "Value"=w99) -> ()  [unwired: 2 in, 2 out]
      n150 = property on="Channel 2" class="Ring (strict)"("Strings []"=w100, "Value"=w99) -> ()  [unwired: 2 in, 2 out]
      n151 = property on="Access" class="Bool (strict)"(error in=w106, "Visible"=w104) -> (error out=w108:errorcluster)  [unwired: 1 in, 1 out]
      n152 = call "Host - Watchdog Init (SubVI).vi"("error in"=w108, "Pilot"=w104) -> ("error out"=w109:errorcluster)  [unwired: 9 in]
      n153 = call "Host Datalog.vi"("Operation"=enum16{"Create", "Write", "Close", "Header"}."Create", "error in"=w109, "Enable"=TRUE) -> ("error out"=w79:errorcluster, "datalog Q"=w102:refnum<queue>)  [unwired: 7 in]
      n154 = Bundle By Name(cluster=w107, "datalog Q"=w102) -> (w81:T30)
      n155 = while {
        tunnel: [w222] -> w89
        tunnel: w79 -> [w221]
        stop <- w223 stop-if-true
        n156 = call "Host Event Log.vi"("Operation"=enum16{"Create", "Write", "Close", "Header"}."Create", "error in"=w221, "Enable"=TRUE) -> ("error out"=w220:errorcluster)  [unwired: 8 in]
        n157 = event shown="[1] \"4K camera P\", \"HD Camera P1\", \"HD Camera P2\", \"HD Camera P3\", \"SD_Camera_P4\", \"LED Light P2\", \"LED Light P3\", \"LED Light P4\", \"4K camera S\", \"HD Camera S1\", \"HD Camera S2\", \"SD Camera S4\", \"HD Camera S3\", \"LED Light S2\", \"LED Light S3\", \"LED Light S4\", \"148 V LED P1\", \"148 V LED P2\", \"148 V LED P3\", \"148 V LED P4\", \"148 V LED S1\", \"148 V LED S2\", \"148 V LED S3\", \"148 V LED S4\", \"Pan and Tilt P1\", \"Pan and Tilt P2\", \"Pan and Tilt S\", \"INS-DVL\", \"Multibeam Sonar\", \"SVP, Turbidity, pH\", \"CO2 Sensor\", \"Trim System\", \"MBS\", \"Methane_Sensor\", \"Laser Light 1\", \"Laser Light 2\", \"Laser Light 3\", \"Laser Light 4\", \"Imaging Sonar\", \"Altimeter\", \"Subbottom Profiler\", \"Magnetometer\", \"Conduct & Temp\", \"Disolved Oxygen\", \"Heat Probe Sensor\", \"Plume Detector\", \"HSSS_P Power\", \"Co2 Scrubber_P\", \"Dehumidifier_P\", \"Co2 Scrubber_S\", \"Dehumidifier_S\", \"VBS SET\", \"HSSS_S Power\", \"Thrusters_T1\", \"Thrusters_T3\", \"Thrusters _T5\", \"Thrusters _T7\", \"Thrusters _T2\", \"Thrusters _T4\", \"Thrusters _T6\", \"Thrusters _T8\", \"T1Power\", \"T2Power\", \"T3Power\", \"T4Power\", \"T5Power\", \"T6Power\", \"T7Power\", \"T1 ctrl\", \"T2 ctrl\", \"T3 ctrl\", \"T4 ctrl\", \"T5 ctrl\", \"T6 ctrl\", \"T7 ctrl\", \"T8 ctrl\", \"T8Power\", \"MBS Freeboard\", \"MBS Desent\", \"MBS_manual\", \"Trim motor enable\", \"VBS_Water out\", \"VBS Water In\", \"Crew Status PILOT\", \"Crew StatusCO-PILOT\", \"Crew Status OBSERVER\": Value Change" {
          selector: _ -> [_ _ _ _ _]
          dyn-events: _ -> [_ _ _ _ _]
          timeout: 100 -> [_ _ _ _ _]
          tunnel: [w227 _ _ TRUE ("Stop?") _] -> w223
          tunnel: [w226 w231 _ _ _] -> w222
          tunnel: w220 -> [w226 _ _ _ _]
          event Timeout {
            n158 = event-data() -> ()  [unwired: 1 in, 1 out]
            n159 = disable-structure shown="Enabled" {
              frame Enabled {
                n160 = call "Host Datalog.vi"("Operation"=enum16{"Create", "Write", "Close", "Header"}."Write", "Enable"=TRUE) -> ()  [unwired: 8 in, 2 out]
              }
              frame Disabled {
              }
            }
            n161 = call "Host - Update Stop.vi"("Operation"=enum16{"Init", "Get", "Set"}."Get") -> ("Stop?"=w227:bool)  [unwired: 9 in, 1 out]
          }
          event "4K camera P", "HD Camera P1", "HD Camera P2", "HD Camera P3", "SD_Camera_P4", "LED Light P2", "LED Light P3", "LED Light P4", "4K camera S", "HD Camera S1", "HD Camera S2", "SD Camera S4", "HD Camera S3", "LED Light S2", "LED Light S3", "LED Light S4", "148 V LED P1", "148 V LED P2", "148 V LED P3", "148 V LED P4", "148 V LED S1", "148 V LED S2", "148 V LED S3", "148 V LED S4", "Pan and Tilt P1", "Pan and Tilt P2", "Pan and Tilt S", "INS-DVL", "Multibeam Sonar", "SVP, Turbidity, pH", "CO2 Sensor", "Trim System", "MBS", "Methane_Sensor", "Laser Light 1", "Laser Light 2", "Laser Light 3", "Laser Light 4", "Imaging Sonar", "Altimeter", "Subbottom Profiler", "Magnetometer", "Conduct & Temp", "Disolved Oxygen", "Heat Probe Sensor", "Plume Detector", "HSSS_P Power", "Co2 Scrubber_P", "Dehumidifier_P", "Co2 Scrubber_S", "Dehumidifier_S", "VBS SET", "HSSS_S Power", "Thrusters_T1", "Thrusters_T3", "Thrusters _T5", "Thrusters _T7", "Thrusters _T2", "Thrusters _T4", "Thrusters _T6", "Thrusters _T8", "T1Power", "T2Power", "T3Power", "T4Power", "T5Power", "T6Power", "T7Power", "T1 ctrl", "T2 ctrl", "T3 ctrl", "T4 ctrl", "T5 ctrl", "T6 ctrl", "T7 ctrl", "T8 ctrl", "T8Power", "MBS Freeboard", "MBS Desent", "MBS_manual", "Trim motor enable", "VBS_Water out", "VBS Water In", "Crew Status PILOT", "Crew StatusCO-PILOT", "Crew Status OBSERVER": Value Change {
            n162 = event-data() -> ("CtlRef"=w235:refnum<vi>, "OldVal"=w234:variant, "NewVal"=w233:variant)  [unwired: 1 in]
            n163 = call "Host - Activity Event Log.vi"("Tab Control"="Tab Control", "NewVal"=w233, "OldVal"=w234, "Control in"=w235) -> ("error out"=w231:errorcluster, "Event"=→"Event Logging":string[][])  [unwired: 6 in]
          }
          event "Mode": Value Change {
            n164 = event-data() -> ("NewVal"=w240:bool)  [unwired: 1 in]
            n165 = case shown="False" w240 {
              tunnel: [u32 0 ("BG Color") u32 16448250 ("BG Color")] -> w238
              tunnel: [w243 w255] -> w239
              tunnel: [u32 7171459 ("Text Color") u32 15202559 ("Text Color")] -> w236
              frame True {
                w243 = u32 16448250 ("Text Color")
                n166 = for {
                  N: 6 -> [_]
                  tunnel: w243 -> [w246]
                  i -> [w247]
                  n167 = case shown="5" w247 {
                    tunnel: w246 -> [w248 w249 w250 w251 w252 w253]
                    frame 0, Default {
                      n168 = property on="Numeric Indicator" class="DigNum (strict)"("NumText.TextColor"=w248) -> ()  [unwired: 2 in, 2 out]
                      n169 = property on="Numeric Indicator" class="DigNum (strict)"("NumText.TextColor"=w248) -> ()  [unwired: 2 in, 2 out]
                    }
                    frame 1 {
                      n170 = property on="Numeric Indicator" class="DigNum (strict)"("NumText.TextColor"=w249) -> ()  [unwired: 2 in, 2 out]
                      n171 = property class="DigNum (strict)"("NumText.TextColor"=w249) -> ()  [unwired: 2 in, 2 out]
                    }
                    frame 2 {
                      n172 = property on="Numeric Indicator" class="DigNum (strict)"("NumText.TextColor"=w250) -> ()  [unwired: 2 in, 2 out]
                      n173 = property on="Numeric Indicator" class="DigNum (strict)"("NumText.TextColor"=w250) -> ()  [unwired: 2 in, 2 out]
                    }
                    frame 3 {
                      n174 = property on="Numeric Indicator" class="DigNum (strict)"("NumText.TextColor"=w251) -> ()  [unwired: 2 in, 2 out]
                      n175 = property on="Numeric Indicator" class="DigNum (strict)"("NumText.TextColor"=w251) -> ()  [unwired: 2 in, 2 out]
                    }
                    frame 4 {
                      n176 = property on="Numeric Indicator" class="DigNum (strict)"("NumText.TextColor"=w252) -> ()  [unwired: 2 in, 2 out]
                      n177 = property on="Numeric Indicator" class="DigNum (strict)"("NumText.TextColor"=w252) -> ()  [unwired: 2 in, 2 out]
                    }
                    frame 5 {
                      n178 = property on="Numeric Indicator" class="DigNum (strict)"("NumText.TextColor"=w253) -> ()  [unwired: 2 in, 2 out]
                      n179 = property on="Numeric Indicator" class="DigNum (strict)"("NumText.TextColor"=w253) -> ()  [unwired: 2 in, 2 out]
                    }
                  }
                }
              }
              frame False {
                w255 = u32 0 ("Text Color")
                n180 = for {
                  N: 4 -> [_]
                  tunnel: w255 -> [w258]
                  i -> [w259]
                  n181 = case shown="0, Default" w259 {
                    tunnel: w258 -> [w260 w261 w262 w263]
                    frame 0, Default {
                      n182 = property on="Numeric Indicator" class="DigNum (strict)"("NumText.TextColor"=w260) -> ()  [unwired: 2 in, 2 out]
                      n183 = property on="Numeric Indicator" class="DigNum (strict)"("NumText.TextColor"=w260) -> ()  [unwired: 2 in, 2 out]
                      n184 = property on="Numeric Indicator" class="DigNum (strict)"("NumText.TextColor"=w260) -> ()  [unwired: 2 in, 2 out]
                    }
                    frame 1 {
                      n185 = property on="Numeric Indicator" class="DigNum (strict)"("NumText.TextColor"=w261) -> ()  [unwired: 2 in, 2 out]
                      n186 = property class="DigNum (strict)"("NumText.TextColor"=w261) -> ()  [unwired: 2 in, 2 out]
                      n187 = property on="Numeric Indicator" class="DigNum (strict)"("NumText.TextColor"=w261) -> ()  [unwired: 2 in, 2 out]
                    }
                    frame 2 {
                      n188 = property on="Numeric Indicator" class="DigNum (strict)"("NumText.TextColor"=w262) -> ()  [unwired: 2 in, 2 out]
                      n189 = property on="Numeric Indicator" class="DigNum (strict)"("NumText.TextColor"=w262) -> ()  [unwired: 2 in, 2 out]
                      n190 = property on="Numeric Indicator" class="DigNum (strict)"("NumText.TextColor"=w262) -> ()  [unwired: 2 in, 2 out]
                    }
                    frame 3 {
                      n191 = property on="Numeric Indicator" class="DigNum (strict)"("NumText.TextColor"=w263) -> ()  [unwired: 2 in, 2 out]
                      n192 = property on="Numeric Indicator" class="DigNum (strict)"("NumText.TextColor"=w263) -> ()  [unwired: 2 in, 2 out]
                      n193 = property on="Numeric Indicator" class="DigNum (strict)"("NumText.TextColor"=w263) -> ()  [unwired: 2 in, 2 out]
                    }
                  }
                }
              }
            }
            n194 = control-ref of="Tab Control"() -> (w241:refnum<vi>)
            n195 = call "Host - Mode Colour change.vi"("Text Color"=w239, "BG Color"=w238, "TabControl in"=w241) -> ()  [unwired: 9 in]
            n196 = control-ref of="Pane"() -> (w237:refnum<vi>)
            n197 = property class="Pane"(reference=w237, "PaneColor"=w236) -> ()  [unwired: 1 in, 2 out]
          }
          event "Quit": Value Change {
            n198 = event-data() -> ()  [unwired: 1 in, 1 out]
            n199 = local read "T7 ctrl"() -> (w272:dbl)
            n200 = local read "T5 ctrl"() -> (w271:dbl)
            n201 = local read "T3 ctrl"() -> (w270:dbl)
            n202 = local read "T1 ctrl"() -> (w269:dbl)
            n203 = local read "T8 ctrl"() -> (w268:dbl)
            n204 = local read "T6 ctrl"() -> (w267:dbl)
            n205 = local read "T4 ctrl"() -> (w266:dbl)
            n206 = local read "T2 ctrl"() -> (w265:dbl)
            n207 = Replace Array Subset(array=dbl[] [0.0, 0.0, 0.0, 0.0, 0.0, 0.0, 0.0, 0.0] ("appended array"), new element #1=w272, new element #2=w271, new element #3=w270, new element #4=w269, new element #5=w268, new element #6=w267, new element #7=w266, new element #8=w265) -> (w264:dbl[])  [unwired: 8 in]
            n208 = for {
              tunnel: [w278] -> w275
              tunnel: w264 -> [w277] mode=indexing
              i -> [w278]
              n209 = for {
                N: w277 -> [w283]
                tunnel: w278 -> [w282]
                i -> [w284]
                n210 = Increment(x=w284) -> (x+1=w279:i32)
                n211 = Subtract(x=w283, y=w279) -> (x-y=w281:i32)
                n212 = case shown="3" w282 {
                  tunnel: w281 -> [w285 w286 w287 w288 w289 w290 w291 w292]
                  frame 0, Default {
                    n213 = local write "T7 ctrl"(w285) -> ()
                  }
                  frame 1 {
                    n214 = local write "T5 ctrl"(w286) -> ()
                  }
                  frame 2 {
                    n215 = local write "T3 ctrl"(w287) -> ()
                  }
                  frame 3 {
                    n216 = local write "T1 ctrl"(w288) -> ()
                  }
                  frame 4 {
                    n217 = local write "T8 ctrl"(w289) -> ()
                  }
                  frame 5 {
                    n218 = local write "T6 ctrl"(w290) -> ()
                  }
                  frame 6 {
                    n219 = local write "T4 ctrl"(w291) -> ()
                  }
                  frame 7 {
                    n220 = local write "T2 ctrl"(w292) -> ()
                  }
                }
                n221 = Wait Until Next ms Multiple(millisecond multiple=u32 250) -> ()  [unwired: 1 out]
              }
            }
            n222 = local write "Warnings/Alarms"("Thruster turning Off") -> ()
            n223 = flat-sequence {
              tunnel: w275 -> [_]
              frame #0 {
                w294 = FALSE ("Thrusters _T8")
                n224 = local write "Thrusters _T8"(w294) -> ()
                n225 = local write "Thrusters _T6"(w294) -> ()
                n226 = local write "Thrusters _T4"(w294) -> ()
                n227 = local write "Thrusters _T2"(w294) -> ()
                n228 = local write "Thrusters _T7"(w294) -> ()
                n229 = local write "Thrusters _T5"(w294) -> ()
                n230 = local write "Thrusters_T3"(w294) -> ()
                n231 = local write "Thrusters_T1"(w294) -> ()
                "Quit?" <- TRUE ("Quit?")
              }
            }
          }
          event "Access": Value Change {
            n232 = event-data() -> ()  [unwired: 1 in, 3 out]
            n233 = call "Host Pilot Access (SubVI).vi"("Master"="Access") -> ()  [unwired: 10 in, 1 out]
          }
        }
      }
      n234 = while {
        shift-right: [w156] -> w97
        shift-left: w81 -> [w160]
        shift-right: [w140] -> w80
        shift-left: w79 -> [w193]
        stop <- w194 stop-if-true
        w116 = 4.5
        w145 = T43."Disabled" ("t")
        w144 = T43."Enabled" ("Disabled")
        (unwired) TRUE ("Enable")
        n235 = property on="Dissolved Oxygen" class="Bool (strict)"() -> ("Value"=w149:bool)  [unwired: 2 in, 2 out]
        n236 = property on="Plume Detector" class="Bool (strict)"() -> ("Value"=w148:bool)  [unwired: 2 in, 2 out]
        n237 = property on="Magnetometer" class="Bool (strict)"() -> ("Value"=w154:bool)  [unwired: 2 in, 2 out]
        n238 = property on="Conduct & Temp" class="Bool (strict)"() -> ("Value"=w153:bool)  [unwired: 2 in, 2 out]
        n239 = Unbundle By Name(w160) -> ("Thruster Cont"=w159:dbl[])
        n240 = Select(t=w145, s=w148, f=w144) -> (s? t:f=w147:T43)
        n241 = Select(t=w145, s=w149, f=w144) -> (s? t:f=w146:T43)
        n242 = Select(t=w145, s=w153, f=w144) -> (s? t:f=w152:T43)
        n243 = Select(t=w145, s=w154, f=w144) -> (s? t:f=w151:T43)
        n244 = Replace Array Subset(array=w159, new element #1="T2 ctrl", new element #2="T4 ctrl", new element #3="T6 ctrl", new element #4="T8 ctrl", new element #5="T1 ctrl", new element #6="T3 ctrl", new element #7="T5 ctrl", new element #8="T7 ctrl", new element #9="led 1 Dim% (10x)", new element #10="led 2 Dim% (10x)") -> (w163:dbl[])  [unwired: 10 in]
        n245 = property on="Conduct & Temp" class="Bool (strict)"("DisabledEnum"=w151) -> ()  [unwired: 2 in, 2 out]
        n246 = property on="Magnetometer" class="Bool (strict)"("DisabledEnum"=w152) -> ()  [unwired: 2 in, 2 out]
        n247 = property on="Plume Detector" class="Bool (strict)"("DisabledEnum"=w146) -> ()  [unwired: 2 in, 2 out]
        n248 = property on="Dissolved Oxygen" class="Bool (strict)"("DisabledEnum"=w147) -> ()  [unwired: 2 in, 2 out]
        n249 = call "Host - Watchdog Process (SubVI).vi"("error in"=w193, "Thuster Clts"=w163, "Data Cluster in"=w160) -> ("error out"=w192:errorcluster, "System Down?"=→"System Down?":bool, "Slave"=→"Slave":bool, "Data Cluster out"=w191:T30)  [unwired: 5 in]
        n250 = call "Host Access Control (SubVI).vi"("Data Cluster in"=w191) -> ()  [unwired: 11 in]
        n251 = call "Host - Update Data (SubVI).vi"("error in"=w192, "Data in"=w191) -> ("error out"=w128:errorcluster, "# elements in queue"=→"elements in queue":i32, "output cluster"=→"output cluster":T1, "Data out"=w157:T30)  [unwired: 6 in]
        n252 = call "Host - Send Serial CMD (SubVI).vi"("Values"=w163, "Camera Controls"="Camera Controls", "Data Cluster"=w157) -> ()  [unwired: 8 in, 1 out]
        n253 = Unbundle By Name(w157) -> ("PS_P"=→"PS_P 2":T26, "IDE_P"=→"IDE_P 2":T26, "PS_S"=→"PS_S 2":T26, "IDE_S"=w126:T26, "PDE_P"=→"PDE_P 2":T26, "PDE_S"=→"PDE_S 2":T26)
        "IDE_S 2" <- w126
        n254 = Unbundle("Camera Controls") -> ("ZOOM IN"=w138:bool, "ZOOM OUT"=w137:bool, "IRIS OPEN"=w136:bool, "IRIS CLOSE"=w135:bool, "ZOOM OUT 2"=w134:bool, "IRIS CLOSE 2"=w133:bool)  [unwired: 1 out]
        n255 = property on="IDE_S IR  (Kohm)" class="DigNum (strict)"() -> ("Value"=w125:dbl)  [unwired: 2 in, 2 out]
        n256 = Replace Array Subset(array=bool[] [FALSE, FALSE, FALSE, FALSE, FALSE, FALSE], new element #1=w138, new element #2=w137, new element #3=w136, new element #4=w135, new element #5=w134, new element #6=w133) -> (w132:bool[])  [unwired: 6 in]
        n257 = Boolean Array To Number(Boolean array=w132) -> (number=w129:u32)
        n258 = Less Or Equal?(x=w125, y=1000.0) -> (x <= y?=w123:bool)
        n259 = call "camera FGV.vi"("Operation"=enum16{"Init", "Get", "Set"}."Set", "error in"=w128, "camera in"=w129) -> ("error out"=w127:errorcluster)  [unwired: 7 in, 1 out]
        n260 = case shown="False" "Joystick" {
          tunnel: w127 -> [w214 w217]
          tunnel: [w214 w216] -> w178
          frame False {
          }
          frame True {
            n261 = call "Nav Joystick read module.vi"("error in"=w217) -> ("Forward"=w215:dbl, "error out"=w216:errorcluster)  [unwired: 6 in, 2 out]
            n262 = local write "T4 ctrl"(w215) -> ()
            n263 = local write "T6 ctrl"(w215) -> ()
            n264 = local write "T2 ctrl"(w215) -> ()
            n265 = local write "T8 ctrl"(w215) -> ()
          }
        }
        n266 = property on="IDE_S IR Status" class="Bool (strict)"("Value"=w123) -> ()  [unwired: 2 in, 2 out]
        n267 = Unbundle By Name(w157) -> ("PS_P.Serial"=w184:string[][], "PS_S.Serial"=w183:string[][], "IDE_P.Serial"=w182:string[][], "IDE_S.Serial"=w181:string[][], "PDE_P.Serial"=w162:string[][], "PDE_S.Serial"=w161:string[][], "TCP - Serial"=→"TCP - Serial":string[][], "Access Restricted?"=w150:bool)
        n268 = Unbundle By Name(w126) -> ("AI"=w122:dbl[])
        "AI" <- w122
        n269 = Index Array(array=w122, index #1=5 ("index"), index #2=6 ("index")) -> (element #1=w118:dbl, element #2=w117:dbl)
        n270 = call "Update GUI (SubVI).vi"("Data out"=w157) -> ("Data out"=w190:T30)  [unwired: 10 in]
        n271 = Greater?(x=w118, y=w116) -> (0:w114:bool)
        n272 = Greater?(x=w117, y=w116) -> (0:w115:bool)
        n273 = Build Array (concatenate)(w184, w183, w182, w181, w162, w161) -> (→"Serial":string[][])
        n274 = Unbundle By Name(w190) -> ("Data Sets"=w199:dbl[][])
        n275 = Or(x=w114, y=w115) -> (x .or. y?=w119:bool)
        n276 = call "Host - Alarm (SubVI).vi"("error in"=w178, "Data in"=w190) -> ("error out"=w141:errorcluster, "Data out"=w156:T30)  [unwired: 7 in, 1 out]
        n277 = property on="IDE_S Water Leak" class="Bool (strict)"("Value"=w119) -> ()  [unwired: 2 in, 2 out]
        n278 = Index Array(array=w199, index (col) #1="Channel", index (col) #2="Channel 2") -> (element #1=→"Graph 1":dbl[], element #2=→"Graph 2":dbl[])  [unwired: 2 in]
        n279 = call "HOST Serial thruster update.vi"("error in (no error)"=w141, "Data out"=w156) -> ("error out"=w140:errorcluster, "Data out 2"=w155:T30)  [unwired: 8 in]
        n280 = call "Host thruste Control Update.vi"("Data out"=w156) -> ("Data out 2"=w142:T30)  [unwired: 9 in, 1 out]
        n281 = case shown="False" w150 {
          tunnel: w155 -> [_ w213]
          tunnel: w142 -> [_ w208]
          frame False {
          }
          frame True {
            n282 = Unbundle By Name(w213) -> ("PDE_P TH Cont.COM 10"=w212:dbl, "PDE_P TH Cont.COM 11"=w211:dbl, "PDE_P TH Cont.COM 12"=w210:dbl, "PDE_P TH Cont.COM 13"=w209:dbl)
            n283 = Unbundle By Name(w208) -> ("PDE_S TH Cont.COM 10"=w207:dbl, "PDE_S TH Cont.COM 11"=w206:dbl, "PDE_S TH Cont.COM 12"=w205:dbl, "PDE_S TH Cont.COM 13"=w204:dbl)
            n284 = property on="T1 ctrl" class="DigNum (strict)"("Value"=w212) -> ()  [unwired: 2 in, 2 out]
            n285 = property on="T3 ctrl" class="DigNum (strict)"("Value"=w211) -> ()  [unwired: 2 in, 2 out]
            n286 = property on="T5 ctrl" class="DigNum (strict)"("Value"=w210) -> ()  [unwired: 2 in, 2 out]
            n287 = property on="T7 ctrl" class="DigNum (strict)"("Value"=w209) -> ()  [unwired: 2 in, 2 out]
            n288 = property on="T2 ctrl" class="DigNum (strict)"("Value"=w207) -> ()  [unwired: 2 in, 2 out]
            n289 = property on="T4 ctrl" class="DigNum (strict)"("Value"=w206) -> ()  [unwired: 2 in, 2 out]
            n290 = property on="T6 ctrl" class="DigNum (strict)"("Value"=w205) -> ()  [unwired: 2 in, 2 out]
            n291 = property on="T8 ctrl" class="DigNum (strict)"("Value"=w204) -> ()  [unwired: 2 in, 2 out]
          }
        }
        n292 = disable-structure shown="Disabled" {
          frame Disabled {
            n293 = call "Acoustic modem TCPIP.vi"("Enum"=T29."read write state", "lOPP COUNT"=4) -> ("Data Tx/Rx"=→"Data Tx/Rx 2":string)  [unwired: 7 in, 2 out]
          }
          frame Enabled {
          }
        }
        n294 = call "Host - Update Stop.vi"("Operation"=enum16{"Init", "Get", "Set"}."Get") -> ("Stop?"=w194:bool)  [unwired: 9 in, 1 out]
        n295 = Wait Until Next ms Multiple(millisecond multiple=u32 50 ("milliseconds to wait")) -> ()  [unwired: 1 out]
      }
      n296 = call "Host Event Log.vi"("Operation"=enum16{"Create", "Write", "Close", "Header"}."Close", "error in"=w89, "Enable"=TRUE) -> ("error out"=w88:errorcluster)  [unwired: 8 in]
      n297 = call "Host Datalog.vi"("Operation"=enum16{"Create", "Write", "Close", "Header"}."Close", "error in"=w88, "Enable"=TRUE) -> ()  [unwired: 7 in, 2 out]
      n298 = disable-structure shown="Disabled" {
        frame Disabled {
          n299 = call "Acoustic modem TCPIP.vi"("Enum"=T29."TCPIP acoustic stop", "lOPP COUNT"=1) -> ()  [unwired: 7 in, 3 out]
        }
        frame Enabled {
        }
      }
      n300 = call "Host - Watchdog Close (SubVI).vi"("error in"=w80) -> ("error out"=w105:errorcluster)  [unwired: 10 in]
      n301 = call <vilib>:"Clear Errors.vi"("error in (no error)"=w105) -> ("error out"=w103:errorcluster)  [unwired: 5 in, 1 out]
      n302 = call "Stop Clone VIs (SubVI).vi"("error in"=w103, "Data Cluster in"=w97) -> ("error out"=w96:errorcluster)  [unwired: 9 in]
      n303 = control-ref of="This VI"() -> (w111:refnum<vi>)
      n304 = call <vilib>:"Clear Errors.vi"("error in (no error)"=w96) -> ("error out"=w110:errorcluster)  [unwired: 5 in, 1 out]
      n305 = disable-structure shown="RUN_TIME_ENGINE==True" {
        disable-tunnel: w111 -> [w297 _]
        disable-tunnel: w110 -> [w296 _]
        frame condition #0 {
          n306 = invoke class="VI" method="FP.Close"(reference=w297, error in=w296) -> ()  [unwired: 1 in, 3 out]
        }
        frame condition #1 (active) {
        }
      }
    }
    frame Error {
    }
  }
  n307 = control-ref of="Tab Control 2"() -> ()  [unwired: 1 out]
  n308 = call <vilib>:"Application Directory.vi"() -> ("Application Directory"=w11:path)
  n309 = Build Path(base path=w11, name or relative path=path "matsya6k.wrl") -> (appended path=w10:path)
  n310 = call <vilib>:"Load VRML File.vi"("error in"=w1, "Path"=w10) -> ("error out"=w4:errorcluster, "Scene:Read Scene File"=w17:refnum<vi>)  [unwired: 8 in]
  n311 = call <vilib>:"Color Change.vi"("Color"=u32 16448250) -> ("RGBA"=w15:cluster{"R":sgl, "G":sgl, "B":sgl, "A":sgl})  [unwired: 10 in]
  n312 = disable-structure shown="Disabled" {
    disable-tunnel: w5 -> [w301 _]
    frame Disabled {
      # "SERIAL MODEM LOOP"
      n313 = call "Stall Data Flow.vim"("value in"=errorcluster {"status"=FALSE, "code"=0, "source"=""} ("error out"), "milliseconds to wait"=u32 100) -> ("value out"=w299:errorcluster)  [unwired: 1 out]
      n314 = while {
        tunnel: w301 -> [w308]
        tunnel: w299 -> [w302]
        stop <- w303 stop-if-true
        n315 = local read "System Down?"() -> (w306:bool)
        n316 = local read "Slave"() -> (w307:bool)
        n317 = Or(x=w306, y=w307) -> (x .or. y?=w305:bool)
        n318 = case shown="True" w305 {
          tunnel: w302 -> [_ w311]
          tunnel: w308 -> [_ w314]
          frame False {
          }
          frame True {
            # "acoustic communication module"
            n319 = local read "Crew Status OBSERVER"() -> (w320:bool)
            n320 = local read "Crew StatusCO-PILOT"() -> (w321:bool)
            n321 = local read "Crew Status PILOT"() -> (w319:bool)
            n322 = Build Array(w319, w321, w320) -> (w315:bool[])
            n323 = call "Serail Modem.vi"("byte count"="Byte Count", "Write Power Status"="Crew Status OBSERVER 2", "Crew Status"=w315, "WRITE BUTTON"="Read/ Write", "error in (no error)"=w311, "piolet/co-p"=w314) -> ("MCC data out"=w328:T44, "USER STRING"=→"USER STRING":string, "Power  Status"=w313:string, "Data out"=→"Data Out":string, "Data Tx/Rx"=w334:string, "Modem Ready Status"=→"Modem Ready Status":bool, "error in (no error) 2"=→"error in (no error) 2":errorcluster)  [unwired: 7 in]
            "Power  Status" <- w313
            n324 = String Length(string=w334) -> (length=→"length":i32)
            n325 = local write "Data Tx/Rx"(w334) -> ()
            n326 = Unbundle By Name(w328) -> ("Acoustic data"=w327:i32, "LATITUDE"=→"Ship Latitude":sgl, "LONGITUDE"=→"Ship Longitude":sgl, "HEADING"=→"Ship Heading":sgl, "TIME"=→"Ship Time":sgl)
            n327 = Decimal String To Number(string=w313) -> (number=→"Radio Buttons 2":i32)  [unwired: 2 in, 1 out]
            n328 = Number To Boolean Array(number=w327) -> (Boolean array=w331:bool[])
            n329 = Index Array(array=w331) -> (element #1=w330:bool, element #2=w329:bool, element #3=w318:bool, element #4=w317:bool, element #5=w316:bool)  [unwired: 5 in]
            n330 = property on="LED Light S2" class="Bool (strict)"("Value"=w330) -> ()  [unwired: 2 in, 2 out]
            n331 = property on="LED Light P2" class="Bool (strict)"("Value"=w329) -> ()  [unwired: 2 in, 2 out]
            n332 = property on="4K camera S" class="Bool (strict)"("Value"=w318) -> ()  [unwired: 2 in, 2 out]
            n333 = property on="4K camera P" class="Bool (strict)"("Value"=w317) -> ()  [unwired: 2 in, 2 out]
            n334 = property on="HD Camera S1" class="Bool (strict)"("Value"=w316) -> ()  [unwired: 2 in, 2 out]
          }
        }
        n335 = call "Host - Update Stop.vi"("Operation"=enum16{"Init", "Get", "Set"}."Get") -> ("Stop?"=w303:bool)  [unwired: 9 in, 1 out]
      }
    }
    frame Enabled {
    }
  }
  n336 = property on="3D MATSYA" class="SceneGraphDisp (strict)"(error in=w4, "Background Color"=w15) -> (error out=w6:errorcluster)  [unwired: 1 in, 1 out]
  n337 = while {
    tunnel: w17 -> [w358]
    tunnel: w6 -> [w357]
    stop <- w353 stop-if-true
    n338 = local read "S_Longitude"() -> (w345:dbl)
    n339 = local read "S_Latitude"() -> (w346:dbl)
    n340 = local read "S_Depth"() -> (w347:dbl)
    n341 = local read "Altitude"() -> (w348:dbl)
    n342 = local read "S_Heading"() -> (w351:dbl)
    n343 = local read "S_Roll"() -> (w350:dbl)
    n344 = local read "S_Pitch"() -> (w349:dbl)
    n345 = Build Array(w351, w350, w349, w348, w347, w346, w345) -> (w344:dbl[])
    n346 = call "Host - Update Stop.vi"("Operation"=enum16{"Init", "Get", "Set"}."Get") -> ("Stop?"=w353:bool)  [unwired: 9 in, 1 out]
    n347 = call "Host - 3D display.vi"("Heading"=w351, "error in"=w357, "Pitch"=w349, "Roll"=w350, "SceneObject in"=w358) -> ("error out"=→"error out 2":errorcluster, "SceneObject out"=→"3D MATSYA":refnum<vi>)  [unwired: 5 in]
    n348 = call "video overlay FGV.vi"("Operation"=enum16{"Init", "Get", "Set"}."Set", "Video overlay input"=w344) -> ("String"=→"String":string)  [unwired: 9 in]
    n349 = call "Elapsed Time"() -> ("Start Time Text"=→"Mission Start Time":string, "Present Text"=→"Present Time":string, "Elapsed Time Text"=→"Completed Time":string)  [unwired: 12 in, 5 out]
    n350 = local read "Quit?"() -> (w338:bool)
    n351 = Not(x=w338) -> (.not. x?=w340:bool)
    n352 = call "Elapsed Time2"("Reset"=w340, "Auto Reset"=w340) -> ("Time has Elapsed"=w339:bool)  [unwired: 10 in, 7 out]
    n353 = Wait Until Next ms Multiple(millisecond multiple=u32 100 ("milliseconds to wait")) -> ()  [unwired: 1 out]
    n354 = case shown="False" w339 {
      frame False {
      }
      frame True {
        n355 = call "Host - Update Stop.vi"("Operation"=enum16{"Init", "Get", "Set"}."Set", "Stop in"=TRUE) -> ()  [unwired: 8 in, 2 out]
      }
    }
  }
  n356 = while {
    stop <- w364 stop-if-true
    n357 = Wait Until Next ms Multiple(millisecond multiple=u32 50 ("milliseconds to wait")) -> ()  [unwired: 1 out]
    n358 = Bundle("Thrusters_T1"="Thrusters_T1", "Thrusters _T2"="Thrusters _T2", "Thrusters_T3"="Thrusters_T3", "Thrusters _T4"="Thrusters _T4", "Thrusters _T5"="Thrusters _T5", "Thrusters _T6"="Thrusters _T6", "Thrusters _T7"="Thrusters _T7", "Thrusters _T8"="Thrusters _T8") -> (w375:T45)  [unwired: 1 in]
    n359 = call "Host - Thrusters signal Update (SubVI).vi"("Thruster Status"=w375) -> ("Thrusters Signal"=w374:T46)  [unwired: 10 in]
    n360 = Unbundle By Name(w374) -> ("T1 - Signal"=w373:bool, "T2 - Signal"=w372:bool, "T3 - Signal"=w371:bool, "T4 - Signal"=w370:bool, "T5 - Signal"=w369:bool, "T6 - Signal"=w368:bool, "T7 - Signal"=w367:bool, "T8 - Signal"=w366:bool)
    n361 = call "Host - Update Stop.vi"("Operation"=enum16{"Init", "Get", "Set"}."Get") -> ("Stop?"=w364:bool)  [unwired: 9 in, 1 out]
    n362 = local write "T2-Signal"(w372) -> ()
    n363 = local write "T1-Signal"(w373) -> ()
    n364 = local write "T3-Signal"(w371) -> ()
    n365 = local write "T4-Signal"(w370) -> ()
    n366 = local write "T5-Signal"(w369) -> ()
    n367 = local write "T6-Signal"(w368) -> ()
    n368 = local write "T7-Signal"(w367) -> ()
    n369 = local write "T8-Signal"(w366) -> ()
  }
  n370 = disable-structure shown="Enabled" {
    frame Disabled {
      n371 = call "Wago PLC.vi"("error in (no error)"=errorcluster {"status"=FALSE, "code"=0, "source"=""}) -> ("error out"=→"error out 3":errorcluster)  [unwired: 10 in]
    }
    frame Enabled {
    }
  }
